vi "运维调试_采配水V3.vi"() -> ()   [LabVIEW 2016, in "PLC.lvlib"]
uses:
  PLC.lvlib
  <vilib>/Plasmionique/MB Master/MB_Master/MB_Master.lvclass
  <vilib>/Utility/miscctls.llb/LVPointTypeDef.ctl
  <vilib>/Plasmionique/MB Master/MB_Master_Serial/MB_Master_Serial.lvclass
  C:/Program Files (x86)/National Instruments/LabVIEW 2016/vi.lib/Plasmionique/MB Master/MB_Master/MB_Master.lvclass
  <vilib>/Instr/_visa.llb/VISA Configure Serial Port (Instr).vi
  <vilib>/NI/Modbus Library/API/Wrapper/Create TCP Slave.vi
  <vilib>/NI/Modbus Library/API/slave/Modbus Slave.lvclass
  <vilib>/Plasmionique/MB Master/MB Master.lvlib
  <vilib>/ptbypt/NI_PtbyPt.lvlib
  <vilib>/NI/Modbus Library/API/Wrapper/API Main.lvlib
panel:
  out "Registers":u16[](array[numeric])
  out "R124":i16 caption="加标回收配水时间"
  out "R44":i16
  in  "V14":bool
  in  "更新程序":bool
  out "R122":i16 caption="二级自来水清洗时间"
  out "R121":i16 caption="一级自来水清洗时间"
  out "R120":i16 caption="过滤自来水清洗时间"
  out "清洗次数":u16
  out "当前启动泵号":u16(ring) items=["1号泵", "2号泵"]
  out "R116":i16 caption="储水时间"
  in  "R113":u16(ring) caption="水箱储水水体" items=["自来水", "水样"]
  out "R112":i16 caption="二级水样池进样超时"
  in  "R111":u16(ring) caption="采配水型号" items=["常规版本", "高配版本"]
  out "数值 19":dbl
  out "数值 18":dbl
  out "数值 17":dbl
  out "数值 16":dbl
  out "数值 15":dbl
  out "数值 14":dbl
  out "数值 13":dbl
  out "数值 12":dbl
  out "数值 11":dbl
  out "数值 10":dbl
  out "数值 9":dbl
  out "数值 8":dbl
  out "数值 7":dbl
  out "数值 6":dbl
  out "数值 5":dbl
  out "数值 4":dbl
  out "数值 3":dbl
  out "数值 2":dbl
  out "数值":dbl
  in  "R118":u16(ring) caption="是否启用质控" items=["不启用质控", "启用质控"]
  out "压力传感器":dbl format="%#.2f"
  out "R110":i16 caption="过滤装置排液时间"
  in  "M4":bool
  in  "M3":bool
  in  "V13":bool
  in  "V12":bool
  in  "V1-R":bool
  in  "V1-G":bool
  in  "V11":bool
  in  "V10":bool
  in  "V9":bool
  in  "V8":bool
  in  "V7-R":bool
  in  "V7-G":bool
  out "X2":bool caption="X1"
  out "采配水版本号":string
  out "R117":i16 caption="清洗频次设定"
  out "通讯故障":bool
  in  "R100":u16(ring) caption="采水泵工作模式" items=["泵1单泵单管路", "泵2单泵单管路", "潜水泵双泵双管路", "自吸泵双泵双管路"]
  out "X11":bool caption="自来水检测_WA"
  out "X10":bool caption="废液报警_WLA"
  out "X9":bool caption="泵2过载报警_KM2"
  out "X8":bool caption="泵1过载报警_KM1"
  out "X7":bool caption="断电检测_DD"
  out "X6":bool caption="门禁开关_MJ"
  out "X5":bool caption="烟雾检测_YW"
  out "X4":bool caption="浸水检测_SJ"
  out "X3":bool caption="水流开关_JY"
  out "X1":bool
  out "X0":bool caption="采样池液位开关_YE1"
  out "R109":i16 caption="外部反冲洗时间"
  out "集成报警信息":string
  out "R108":i16 caption="进样超时时间"
  out "R107":i16 caption="进气时间"
  out "R106":i16 caption="排液时间"
  out "R105":i16 caption="常规模式配水时间"
  out "R104":i16 caption="过滤次数"
  out "R103":i16 caption="过滤配水时间"
  out "R102":i16 caption="一级沉淀时间"
  out "R101":i16 caption="管路润洗时间"
  out "R2":i16
  out "R1":i16
  out "多列列表框":i32(listbox)
  in  "V6":bool
  in  "V5":bool
  in  "V4":bool
  in  "V3":bool
  in  "V2":bool
  in  "M2":bool
  in  "M1":bool
  in  "返回":bool
  in  "参数设置":bool
  in  "单步启动":bool
  in  "启动":bool
  in  "停止":bool
  # "流程计时："
  # "s"
  # "压力传感器："
  # "MPa"
  # "二级液位开关低_Y2FD"
  # "二级液位开关高_YF2H"
  # "S"
  # "S"
  # "S"
  # "S"
  # "S"
  # "S"
  # "次"
  # "S"
  # "S"
  # "S"
  # "S"
  # "S"
  # "S"
  # "单步计时："
  # "s"
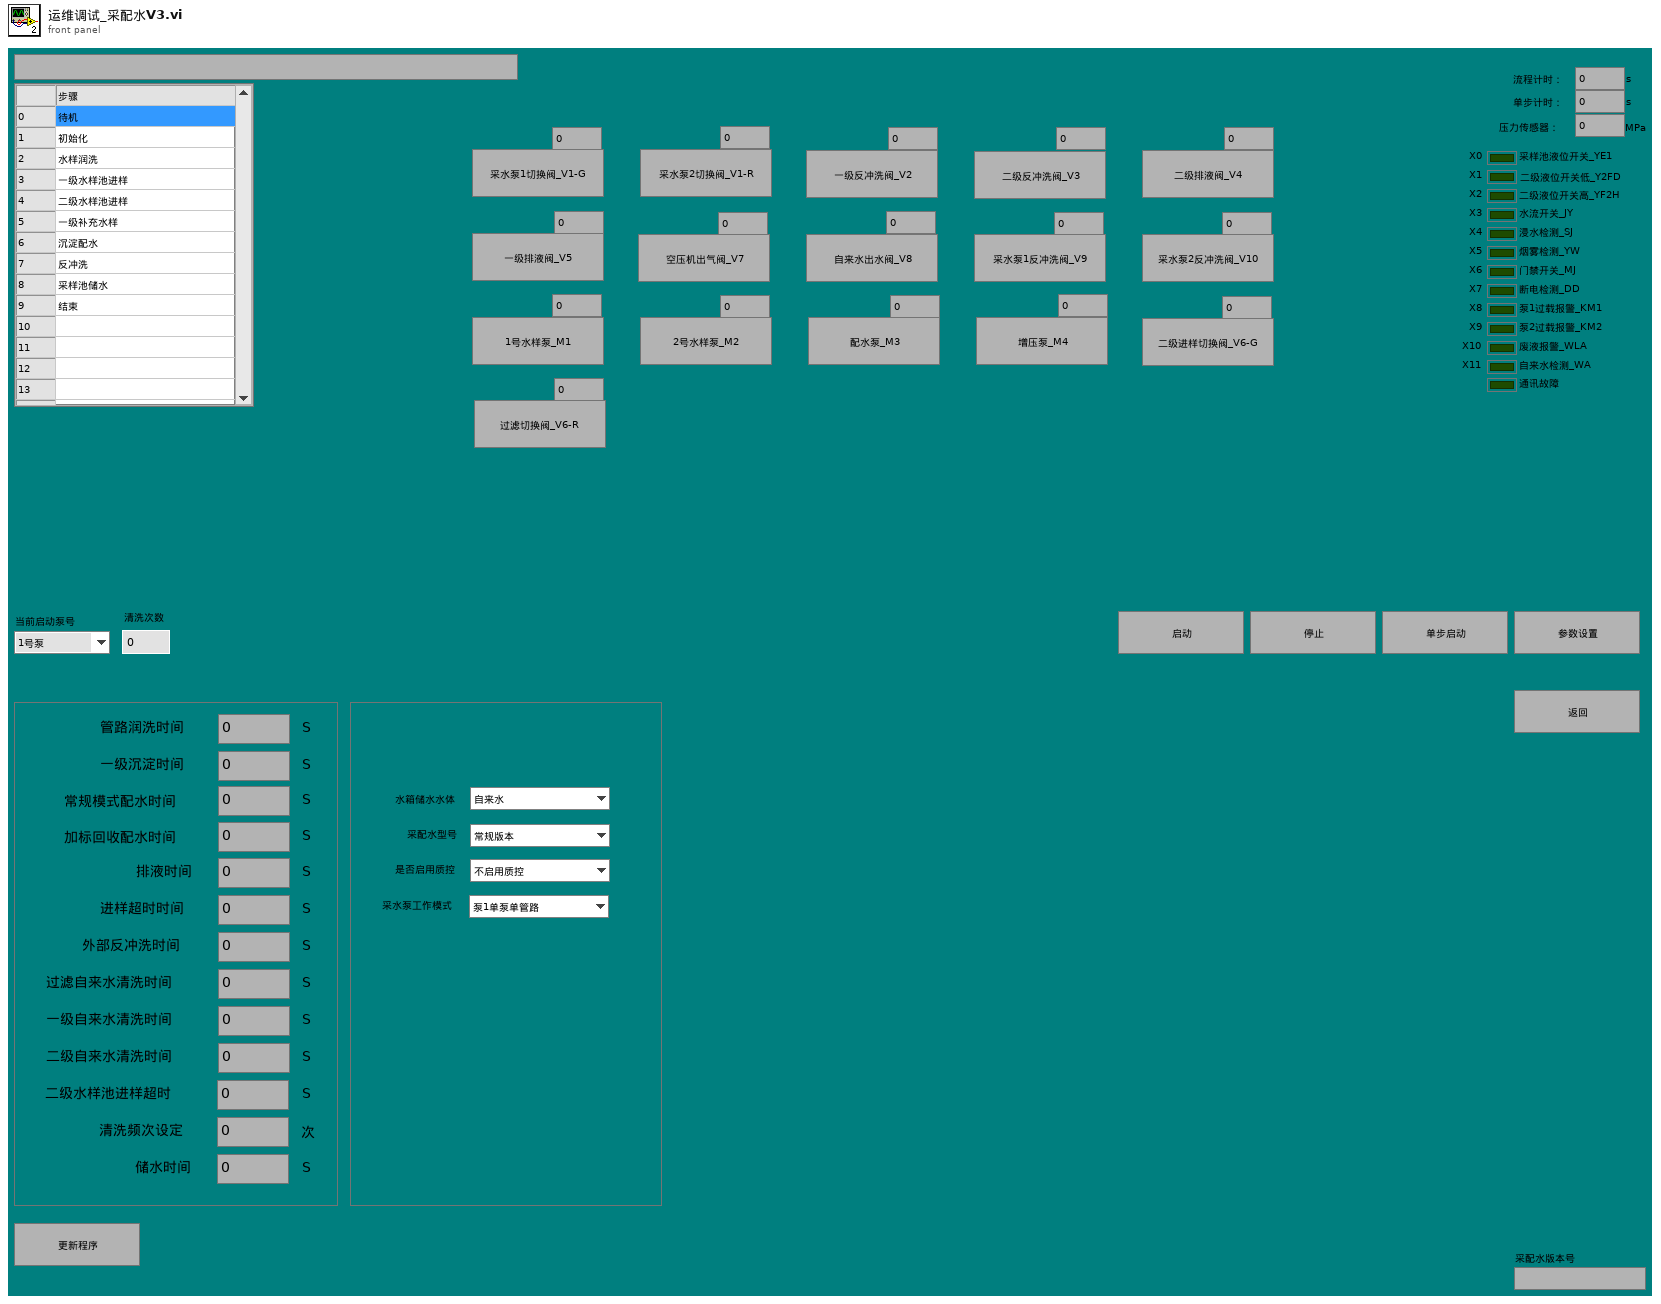
[diagram p1: front panel]
types:
  T1 = typedef "LVPointTypeDef.ctl" = cluster{"Horizontal":i16, "Vertical":i16}
  T2 = cluster{"命令":string, "数据":cluster{"starting address":u16, "holding register value":u16}}
  T3 = cluster{"时间标识":timestamp, "设备":string, "日志信息":string}
  T4 = cluster{"R0":i16, "R1":i16, "R2":i16, "R3":i16, "R4":i16, "R5":i16, "R6":i16, "R7":i16, "R8":i16, "R9":i16, "R10":i16, "R11":i16, "R12":i16, "R13":i16, "R14":i16, "R15":i16, "R16":i16, "R17":i16, "R18":i16, "R19":i16, "R20":i16, "R21":i16, "R22":i16, "R23":i16, "R24":i16, "R25":i16, "R26":i16, "R27":i16, "R28":i16, "R29":i16, "R30":i16, "R31":i16, "R32":i16, "R33":i16, "R34":i16, "R35":i16, "R36":i16, "R37":i16, "R38":i16, "R39":i16, "R40":i16, "R41":i16, "R42":i16, "R43":i16, "R44":i16, "R45":i16, "R46":i16, "R47":i16, "R48":i16, "R49":i16, "R50":i16, "R51":i16, "R52":i16, "R53":i16, "R54":i16, "R55":i16, "R56":i16}
  T5 = cluster{"seconds since 1Jan1904":timestamp, "table输入":string, string, "table输入":string}
  T6 = cluster{"时间标识":timestamp, "设备":string, "日志信息":string, "流程参数":string}
  T7 = cluster{"命令":string, cluster{"starting address":u16, "holding register value":u16}}
  T8 = cluster{"命令":string, "数据":cluster{"starting address":u16, "holding register values":u16[]}}
  T9 = cluster{"命令":string, "data":cluster{"starting address":u16, "coil values":bool[]}}
  T10 = cluster{"测试模式":enum16{"正常测试", "集成干预"}, "参数启用":cluster{"氨氮":bool, "总磷总氮":bool, "CODMn":bool, "CODcr":bool, "多参数":bool, "超标留样":bool, "总氮":bool}}
  T11 = enum32{"Bad", "Idle", "Run top level", "Running"}
  T12 = cluster{"baud rate (bps)":u32, "stop bits":u16, "parity":u16, "flow control":u16, "timeout":u32, "retries":i32}
  T13 = cluster{"starting address":u16, "holding register values":u16[]}
  T14 = cluster{"starting address":u16, "holding register value":u16}
  T15 = cluster{"starting address":u16, "coil values":bool[]}
  T16 = cluster{"Registers[0]":u16, "Registers[1]":u16, "Registers[2]":u16, "Registers[3]":u16, "Registers[4]":u16, "Registers[5]":u16, "Registers[6]":u16, "Registers[7]":u16, "Registers[8]":u16, "Registers[9]":u16, "Registers[10]":u16, "Registers[11]":u16, "Registers[12]":u16, "Registers[13]":u16, "Registers[14]":u16, "Registers[15]":u16, "Registers[16]":u16, "Registers[17]":u16, "Registers[18]":u16, "Registers[19]":u16, "Registers[20]":u16, "Registers[21]":u16, "Registers[22]":u16, "Registers[23]":u16, "Registers[24]":u16, "Registers[25]":u16, "Registers[26]":u16, "Registers[27]":u16, "Registers[28]":u16, "Registers[29]":u16, "Registers[30]":u16, "Registers[31]":u16, "Registers[32]":u16, "Registers[33]":u16, "Registers[34]":u16, "Registers[35]":u16, "Registers[36]":u16, "Registers[37]":u16, "Registers[38]":u16, "Registers[39]":u16, "Registers[40]":u16, "Registers[41]":u16, "Registers[42]":u16, "Registers[43]":u16, "Registers[44]":u16, "Registers[45]":u16, "Registers[46]":u16, "Registers[47]":u16, "Registers[48]":u16, "Registers[49]":u16, "Registers[50]":u16, "Registers[51]":u16, "Registers[52]":u16, "Registers[53]":u16, "Registers[54]":u16, "Registers[55]":u16, "Registers[56]":u16}
  T17 = cluster{"Registers[0]":u16, "Registers[1]":u16, "Registers[2]":u16, "Registers[3]":u16, "Registers[4]":u16, "Registers[5]":u16}
  T18 = cluster{"Registers[0]":u16, "Registers[1]":u16, "Registers[2]":u16, "Registers[3]":u16, "Registers[4]":u16, "Registers[5]":u16, "Registers[6]":u16, "Registers[7]":u16, "Registers[8]":u16, "Registers[9]":u16, "Registers[10]":u16, "Registers[11]":u16, "Registers[12]":u16, "Registers[13]":u16, "Registers[14]":u16, "Registers[15]":u16, "Registers[16]":u16, "Registers[17]":u16, "Registers[18]":u16, "Registers[19]":u16, "Registers[20]":u16, "Registers[21]":u16, "Registers[22]":u16, "Registers[23]":u16, "Registers[24]":u16}
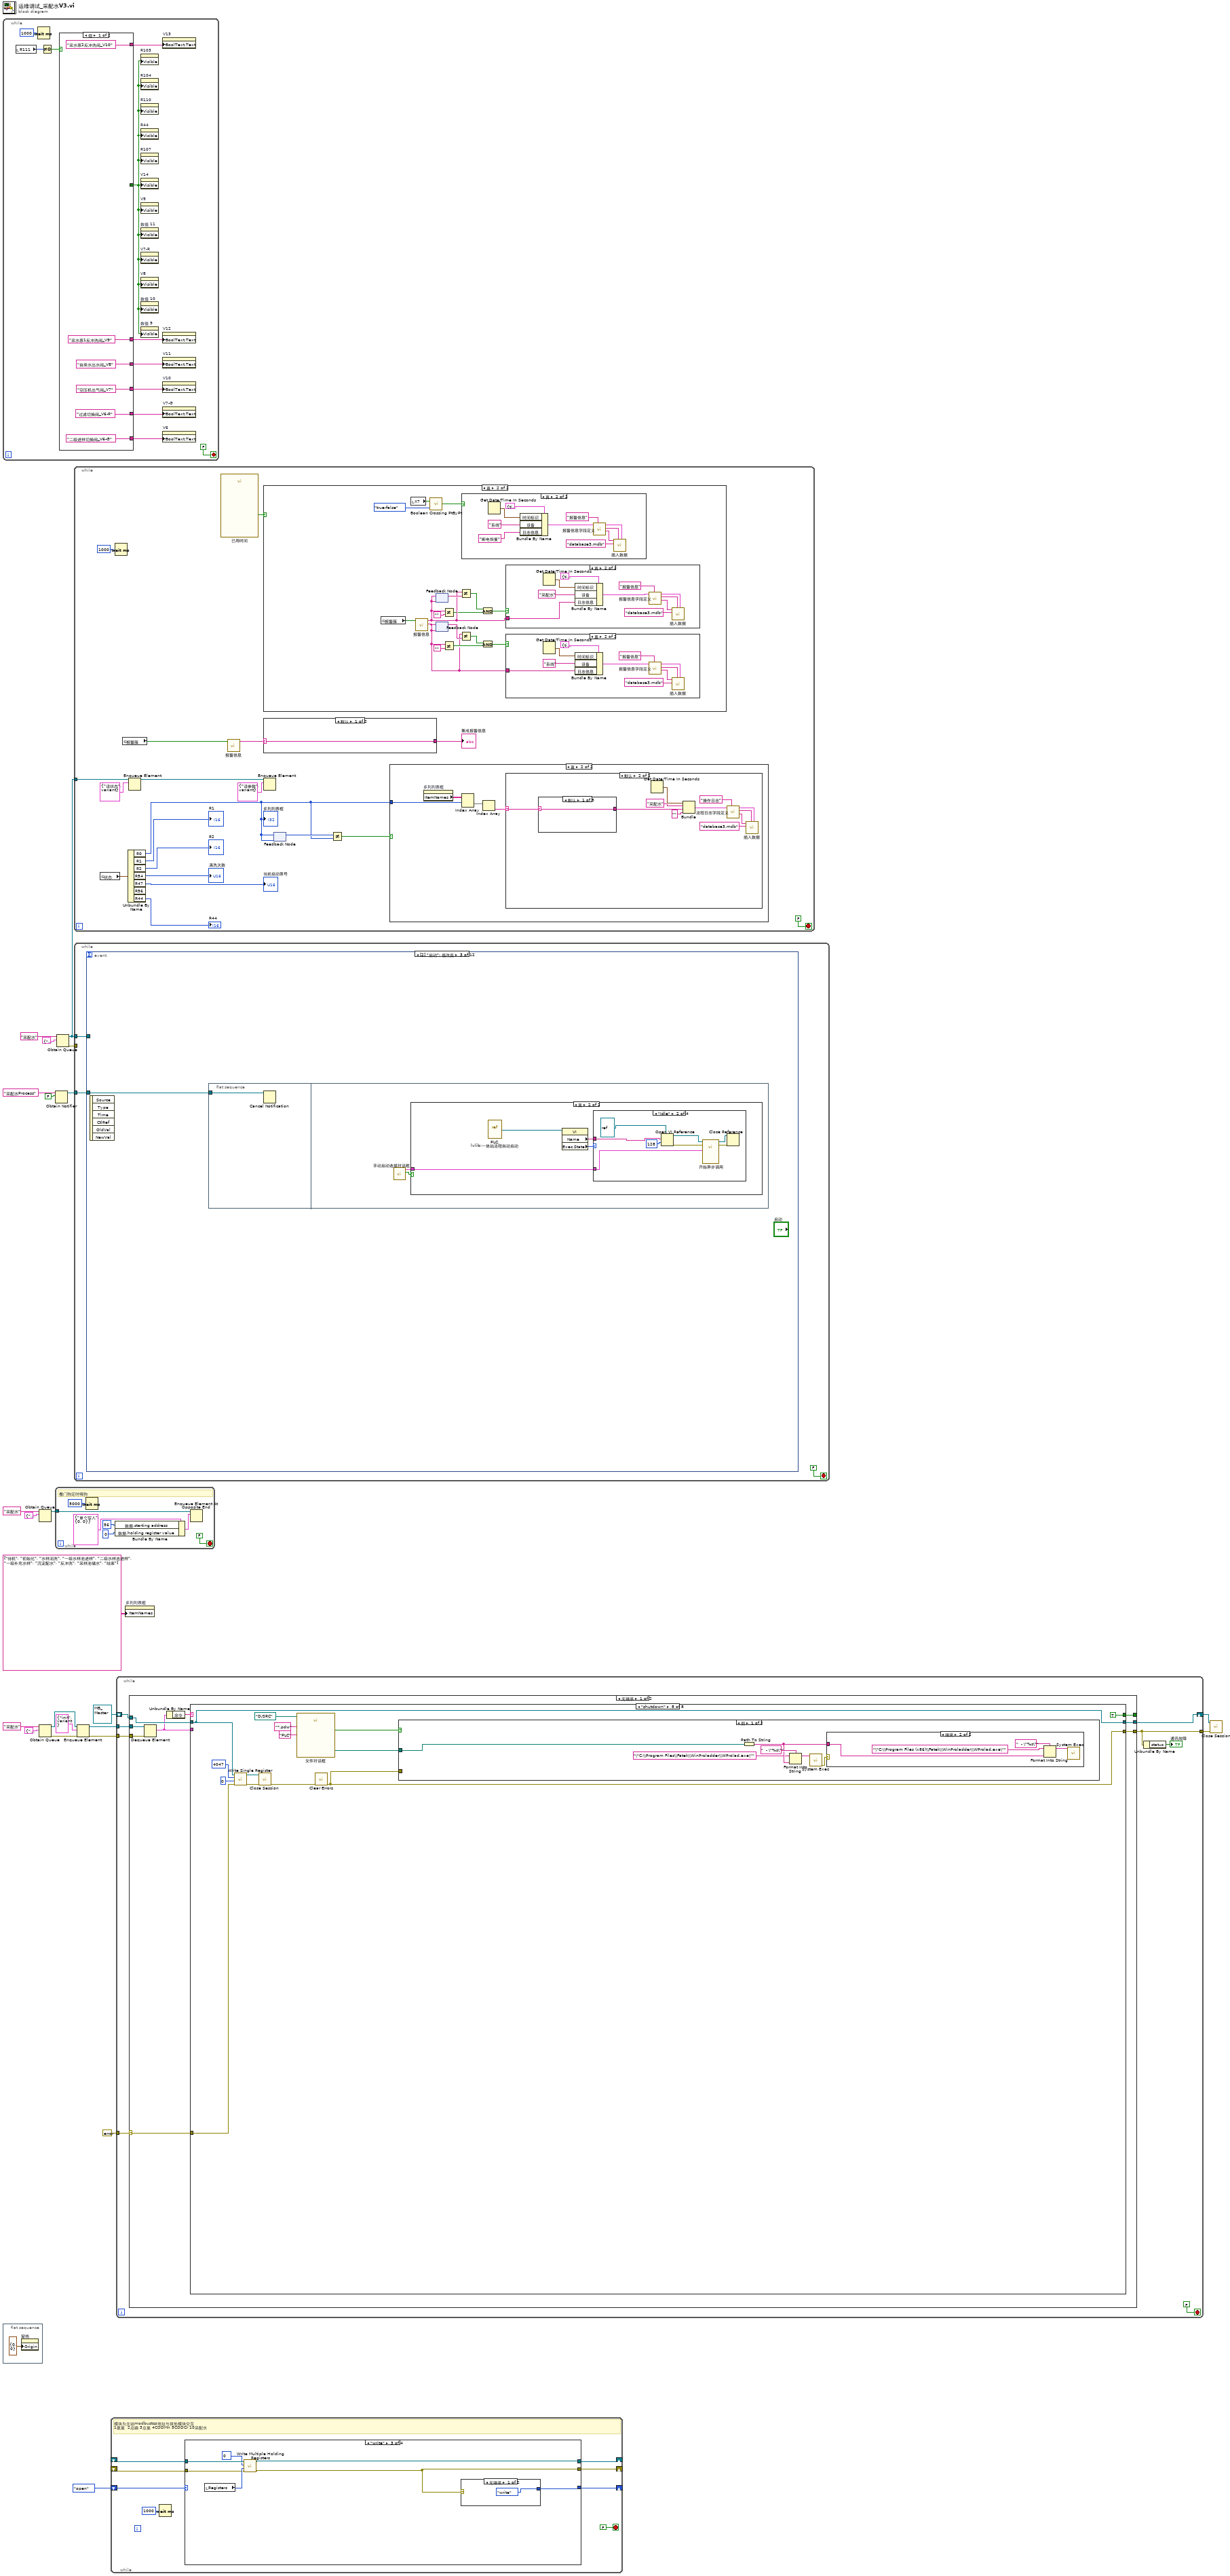
[diagram p0: block diagram]
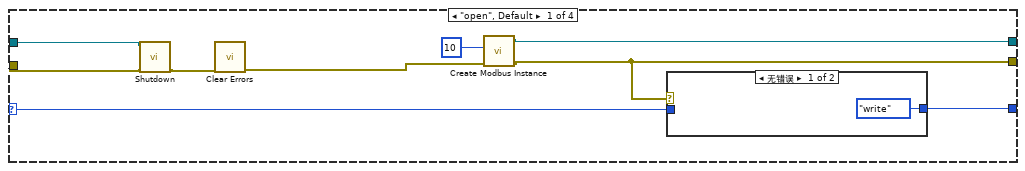
[diagram p2: hidden frame]
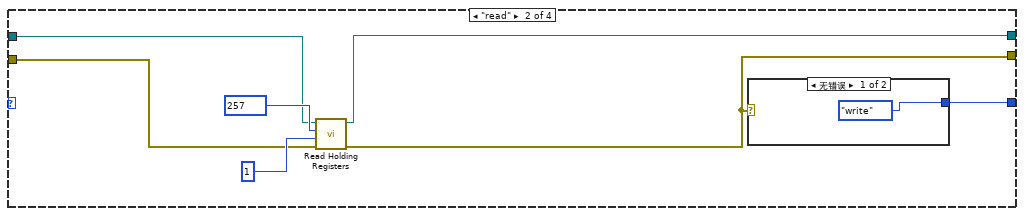
[diagram p4: hidden frame]
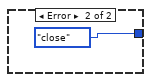
[diagram p5: hidden frame]
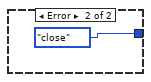
[diagram p6: hidden frame]
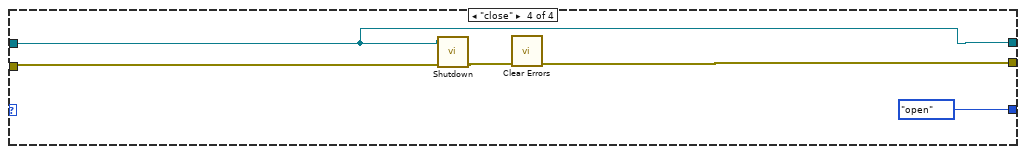
[diagram p7: hidden frame]
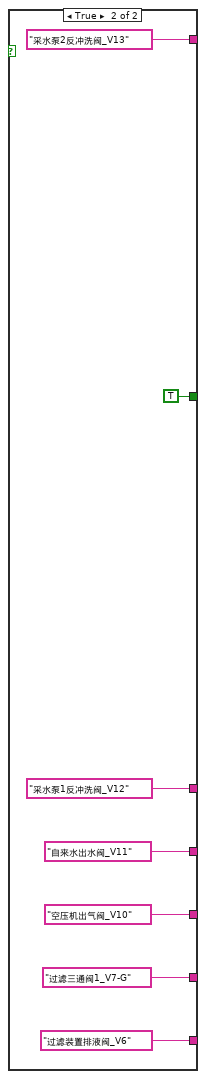
[diagram p8: hidden frame]
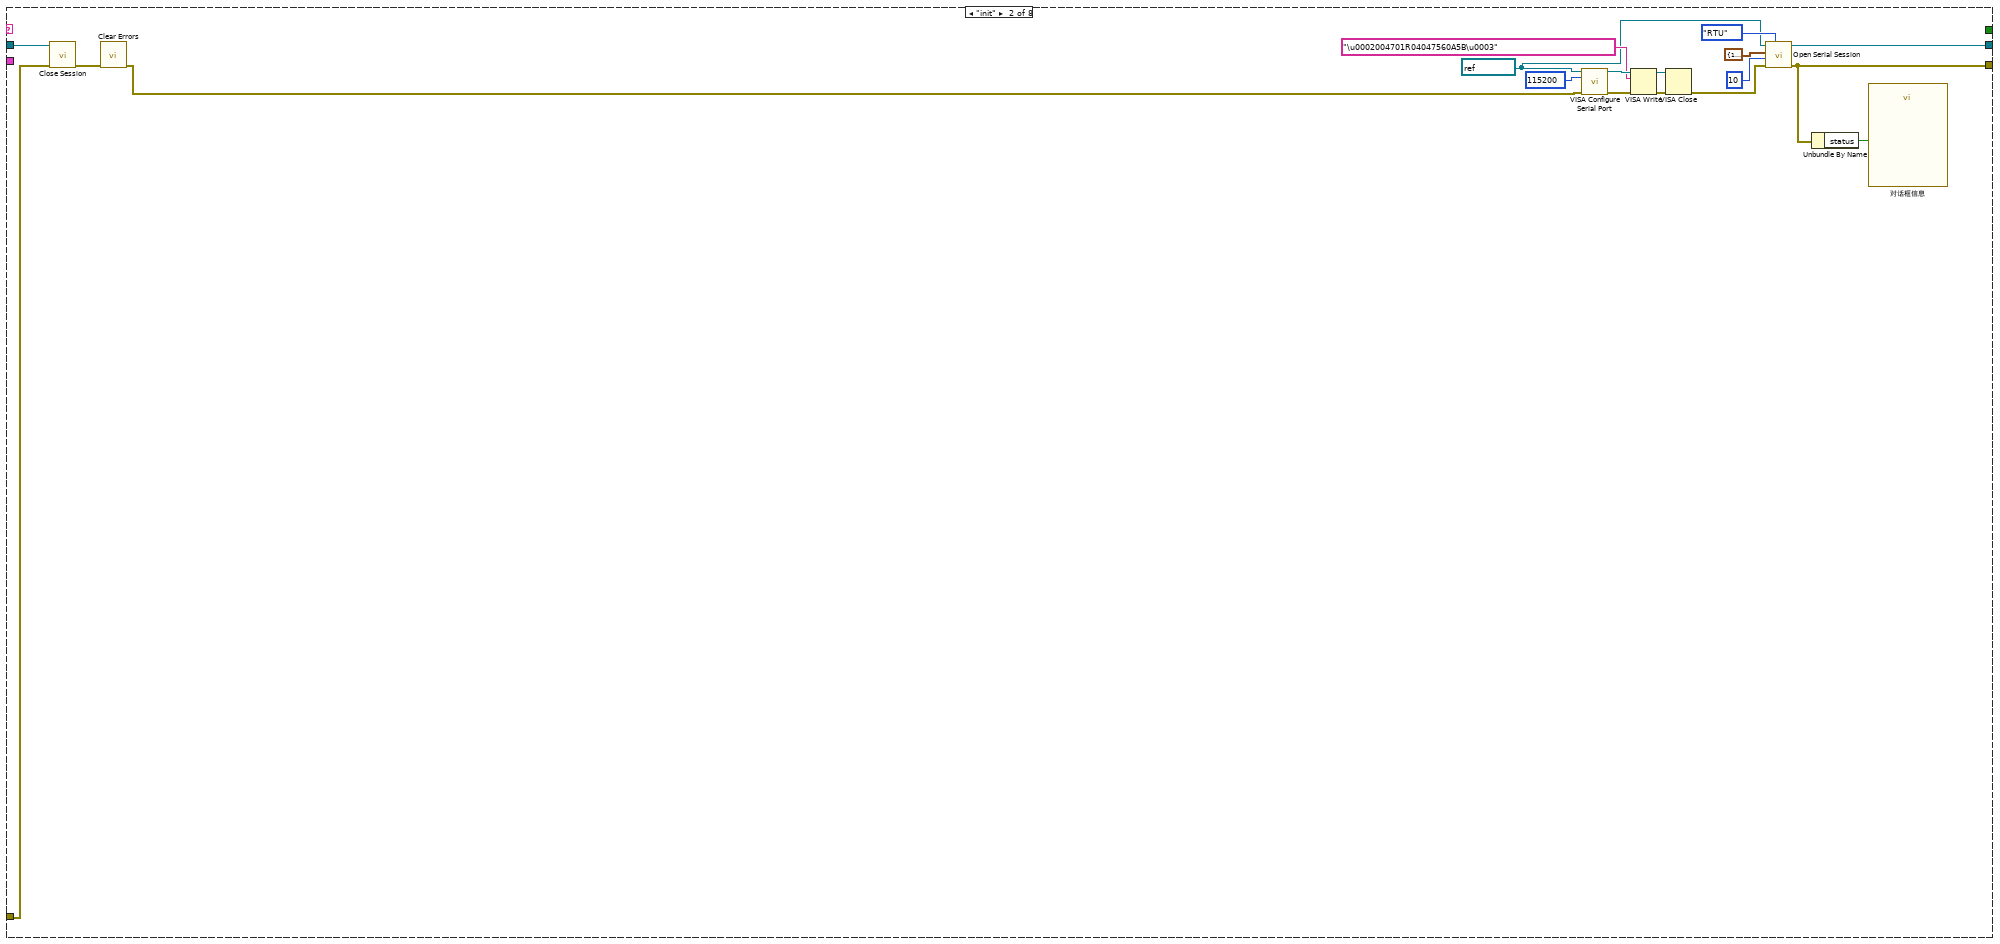
[diagram p10: hidden frame]
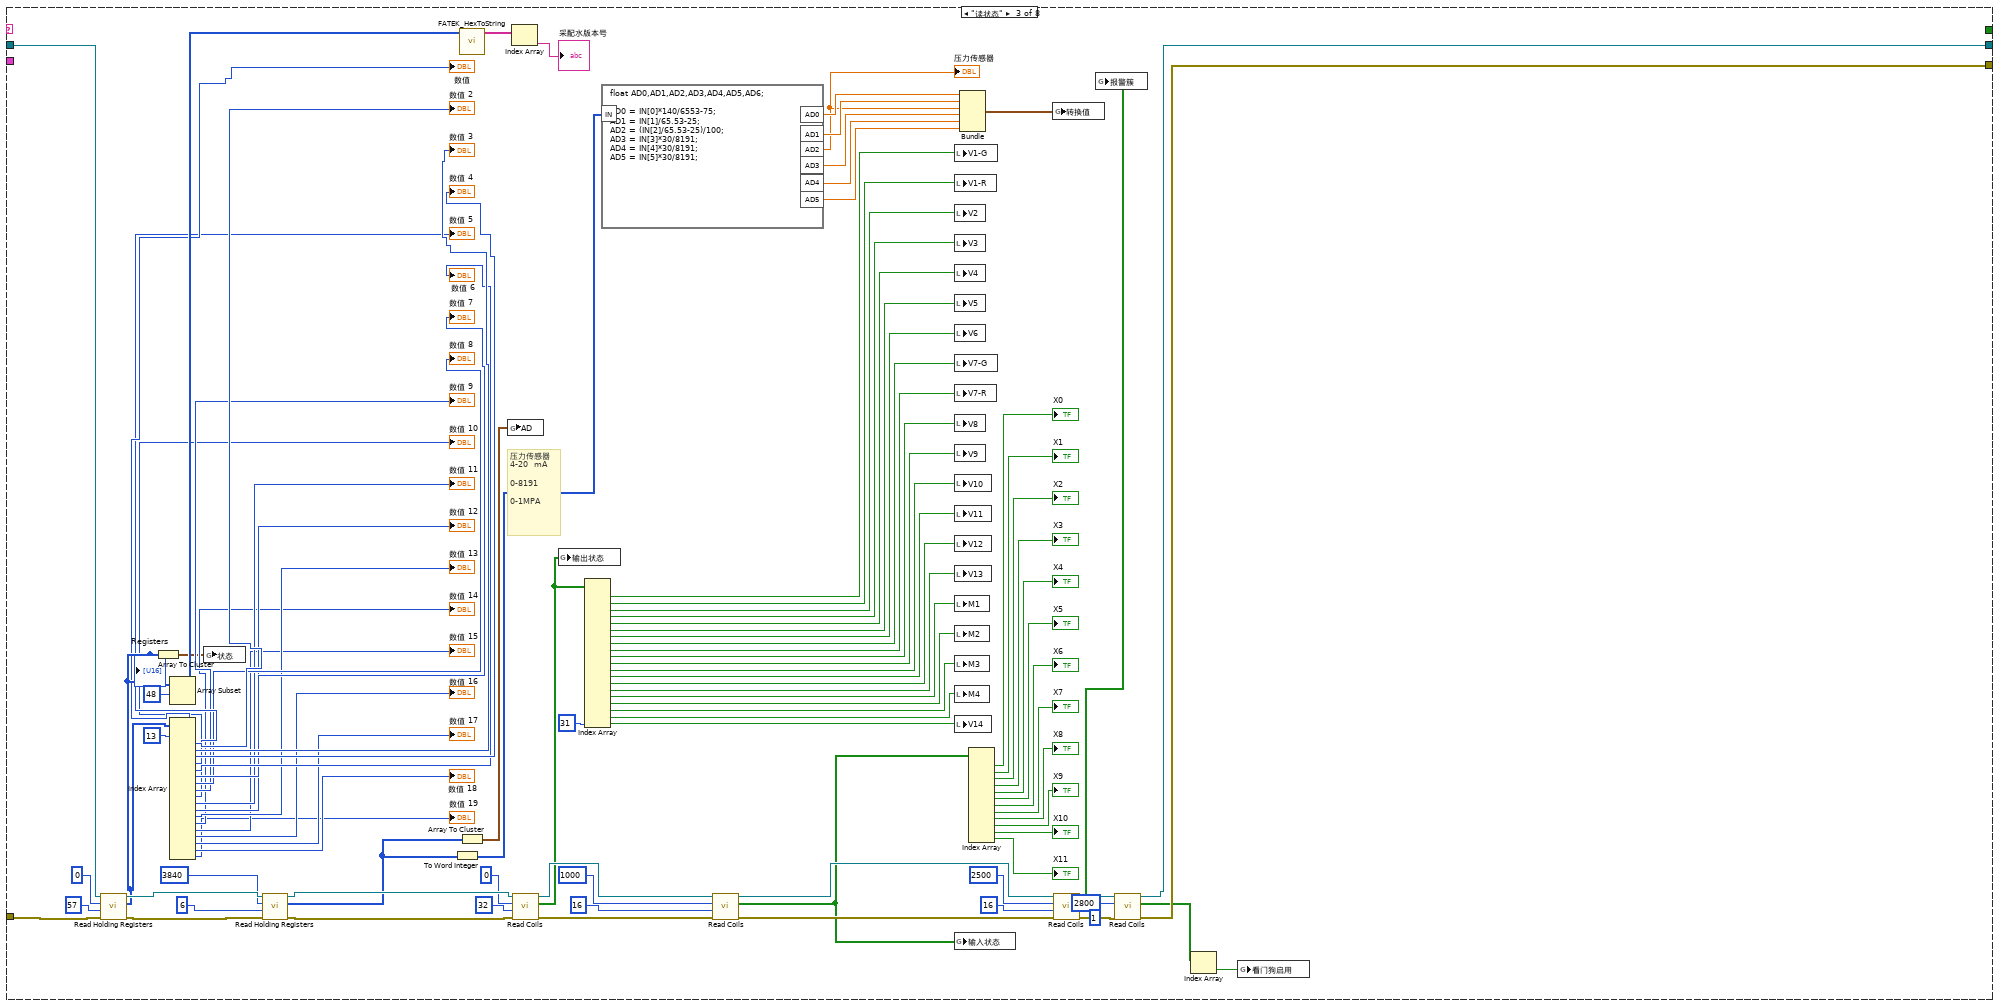
[diagram p11: hidden frame]
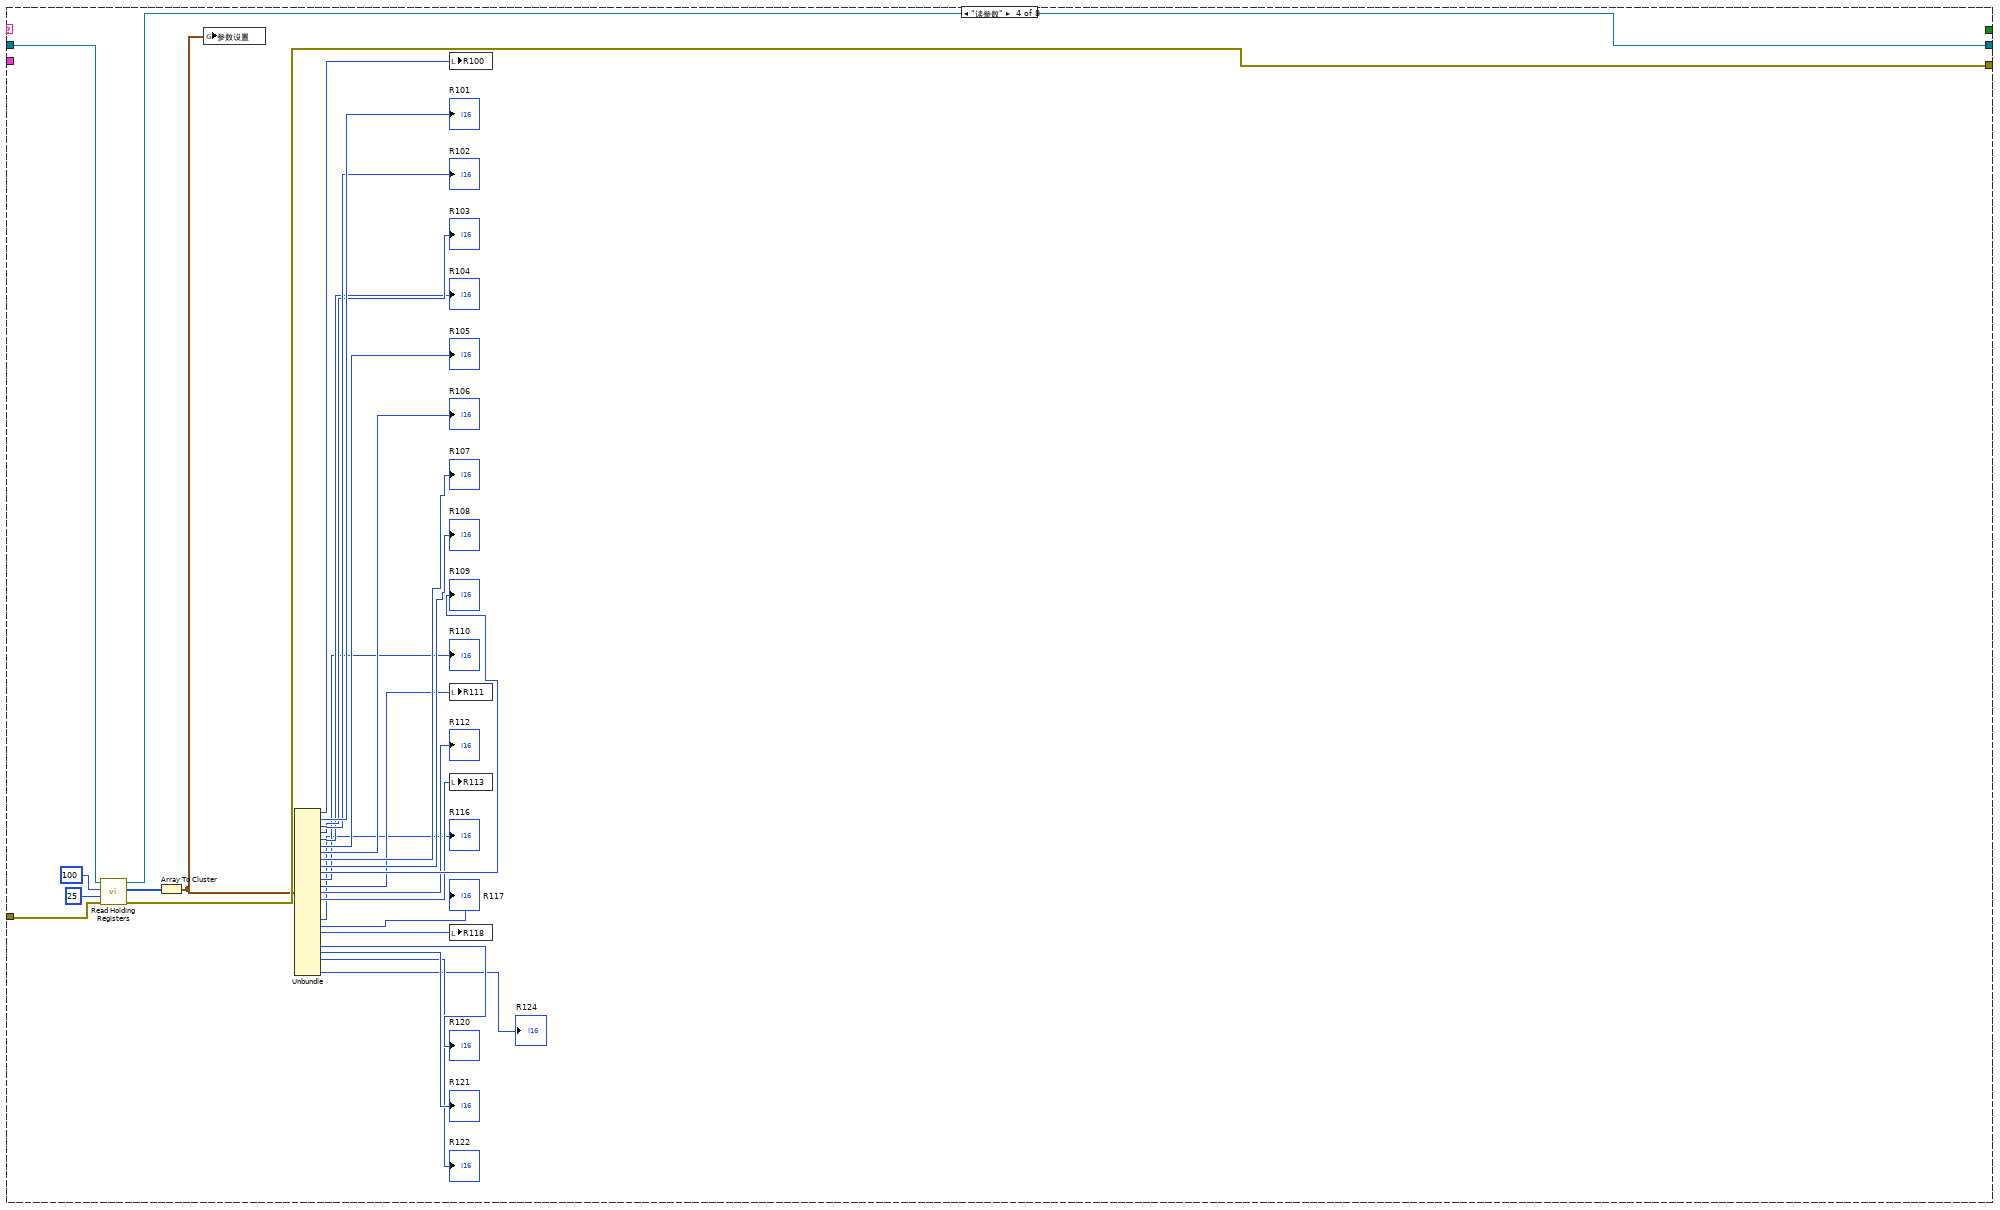
[diagram p12: hidden frame]
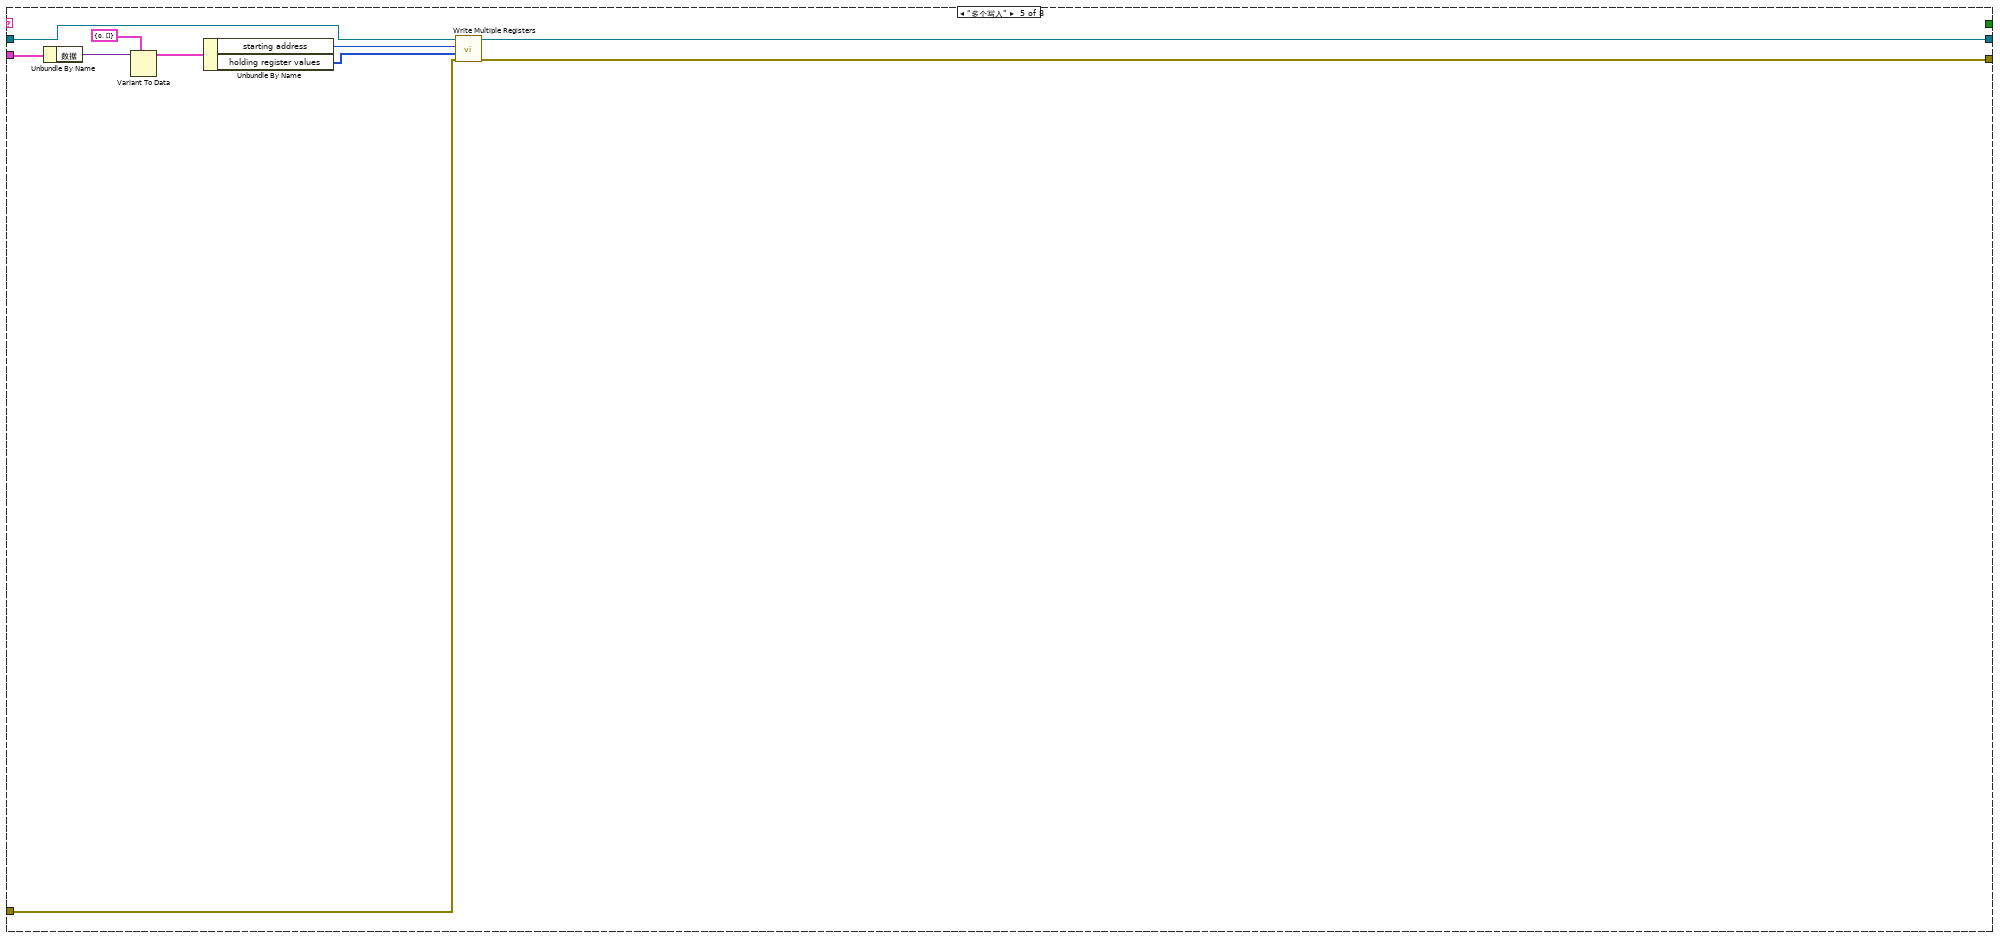
[diagram p13: hidden frame]
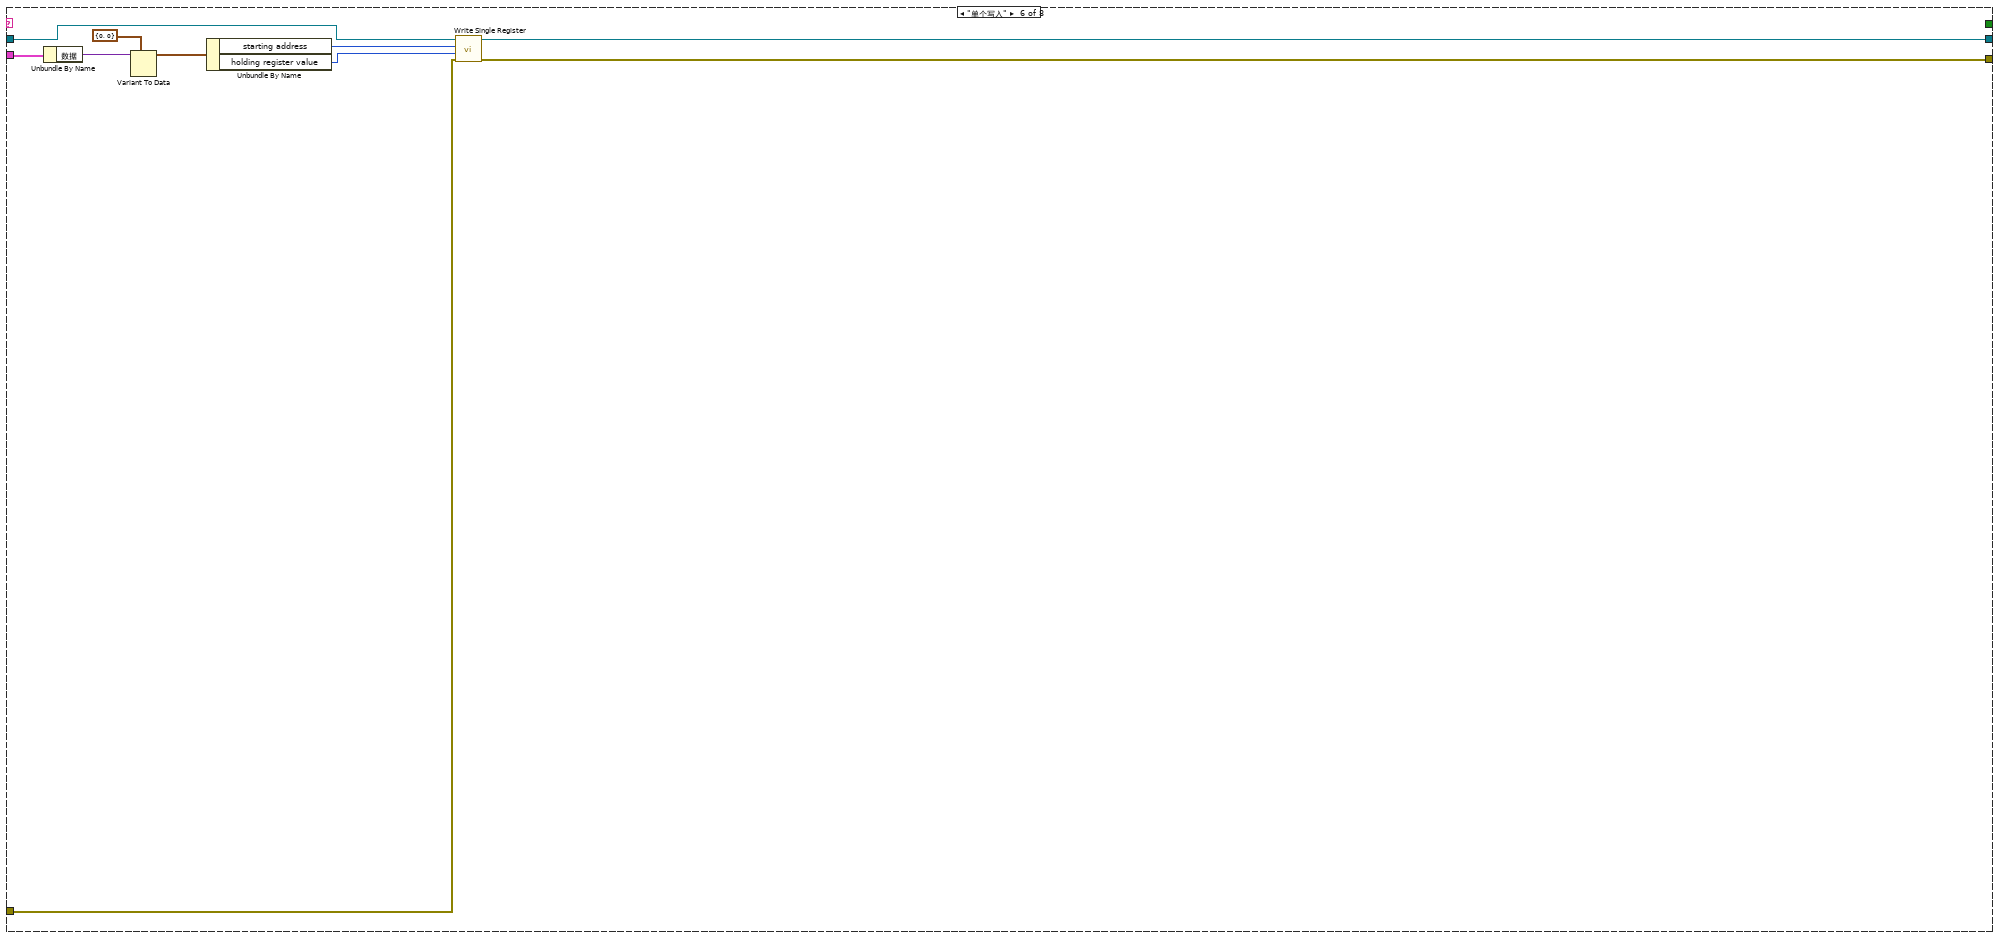
[diagram p14: hidden frame]
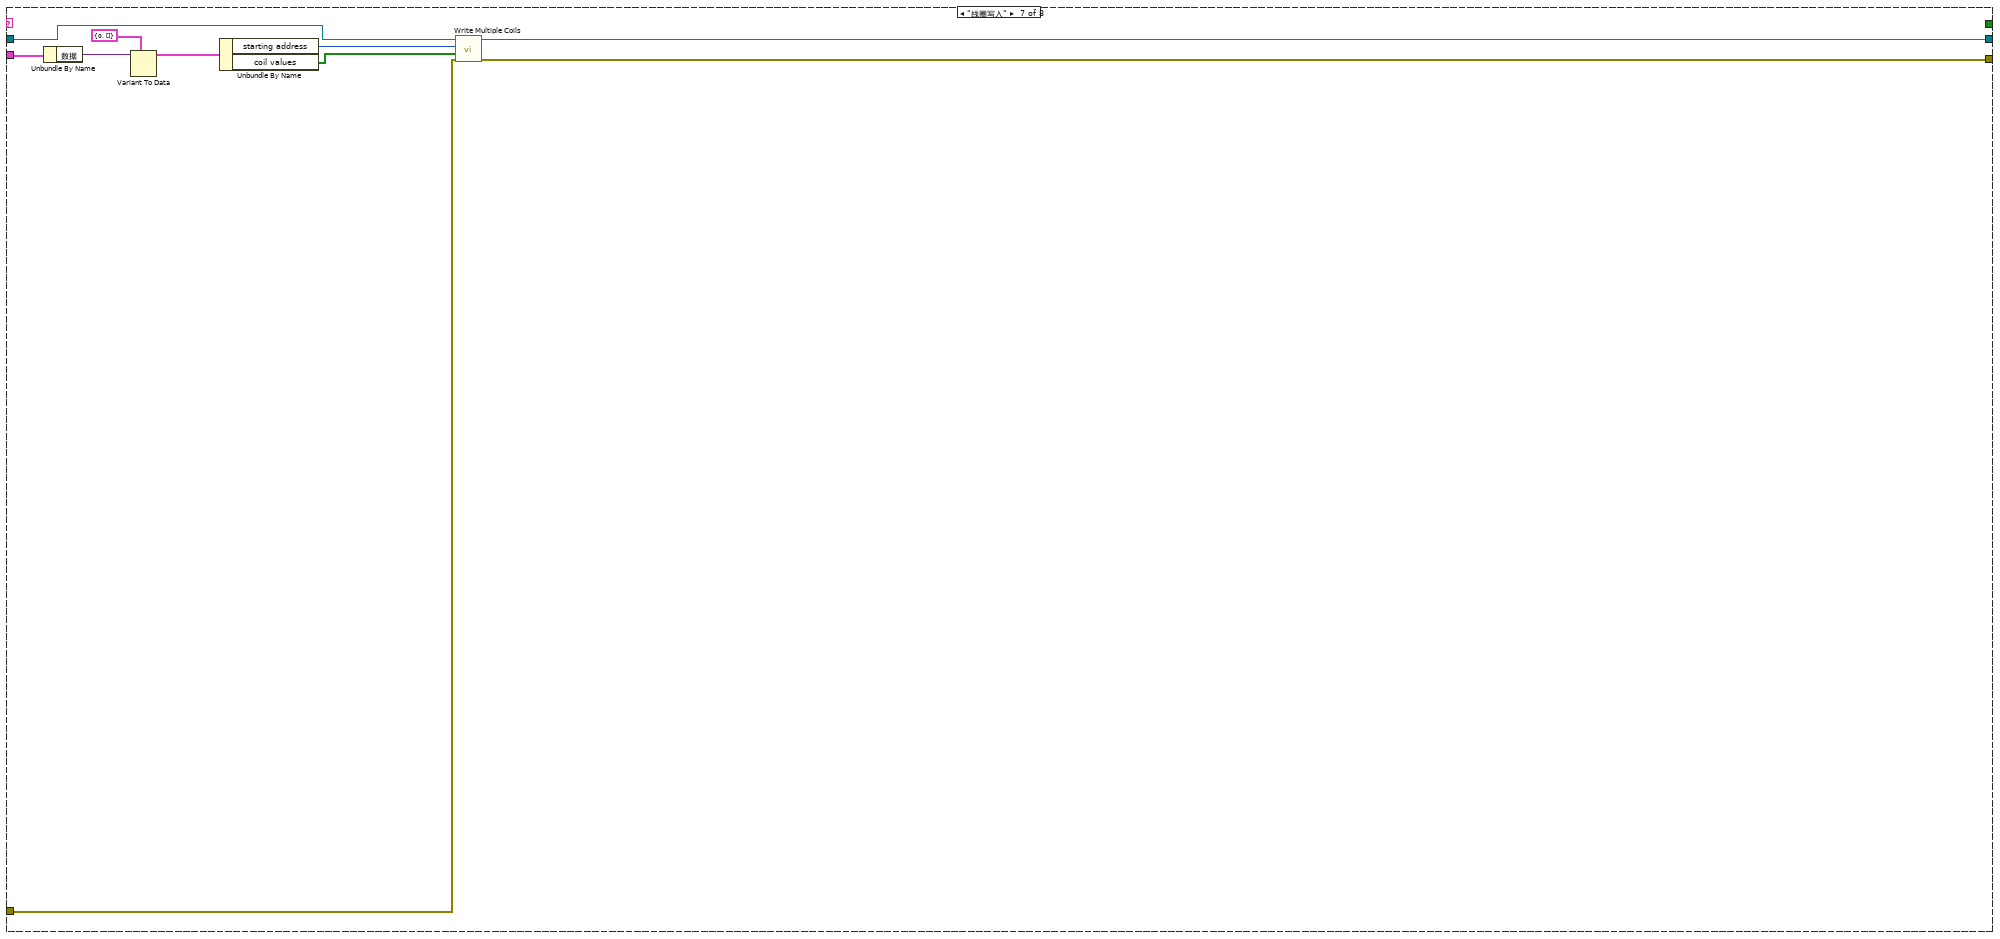
[diagram p15: hidden frame]
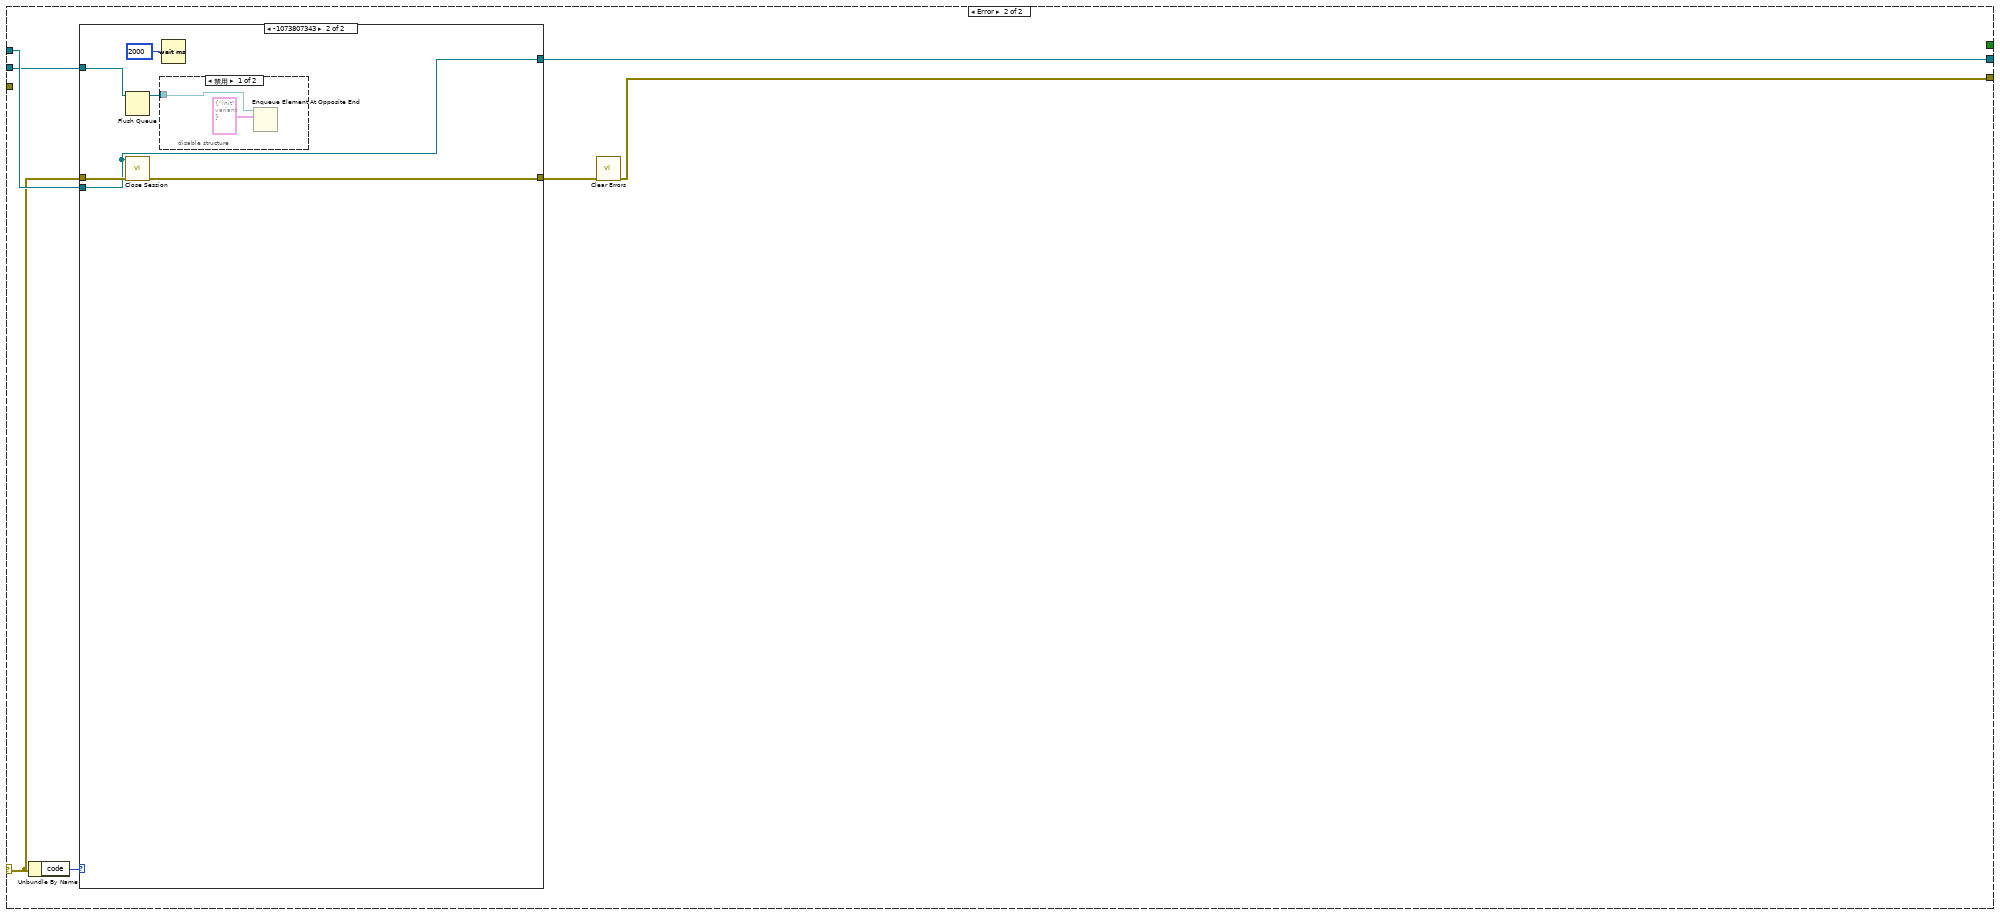
[diagram p18: hidden frame]
diagram:
  n1 = while {
    stop <- FALSE stop-if-true
    n2 = local read "R111"() -> (w33:u16)
    n3 = Wait (ms)(milliseconds to wait=u32 1000 ("等待时间（毫秒）")) -> ()  [unwired: 1 out]
    n4 = Not Equal To 0?(x=w33) -> (x != 0?=w32:bool)
    n5 = case shown="假" w32 {
      tunnel: [_ TRUE ("可见")] -> w24
      tunnel: ["二级进样切换阀_V6-G" ("布尔文本.文本") "过滤装置排液阀_V6" ("布尔文本.文本")] -> w30
      tunnel: ["过滤切换阀_V6-R" ("布尔文本.文本") "过滤三通阀1_V7-G" ("布尔文本.文本")] -> w29
      tunnel: ["空压机出气阀_V7" ("布尔文本.文本") "空压机出气阀_V10" ("布尔文本.文本")] -> w28
      tunnel: ["自来水出水阀_V8" ("布尔文本.文本") "自来水出水阀_V11" ("布尔文本.文本")] -> w27
      tunnel: ["采水泵1反冲洗阀_V9" ("布尔文本.文本") "采水泵1反冲洗阀_V12" ("布尔文本.文本")] -> w26
      tunnel: ["采水泵2反冲洗阀_V10" ("布尔文本.文本") "采水泵2反冲洗阀_V13" ("布尔文本.文本")] -> w25
      frame False {
      }
      frame True {
      }
    }
    n6 = property on="R103" class="DigNum (严格)"("Visible"=w24) -> ()  [unwired: 2 in, 2 out]
    n7 = property on="R104" class="DigNum (严格)"("Visible"=w24) -> ()  [unwired: 2 in, 2 out]
    n8 = property on="R110" class="DigNum (严格)"("Visible"=w24) -> ()  [unwired: 2 in, 2 out]
    n9 = property on="R44" class="DigNum (严格)"("Visible"=w24) -> ()  [unwired: 2 in, 2 out]
    n10 = property on="R107" class="DigNum (严格)"("Visible"=w24) -> ()  [unwired: 2 in, 2 out]
    n11 = property on="V14" class="Bool (严格)"("Visible"=w24) -> ()  [unwired: 2 in, 2 out]
    n12 = property on="V9" class="Bool (严格)"("Visible"=w24) -> ()  [unwired: 2 in, 2 out]
    n13 = property on="数值 11" class="DigNum (严格)"("Visible"=w24) -> ()  [unwired: 2 in, 2 out]
    n14 = property on="V7-R" class="Bool (严格)"("Visible"=w24) -> ()  [unwired: 2 in, 2 out]
    n15 = property on="V8" class="Bool (严格)"("Visible"=w24) -> ()  [unwired: 2 in, 2 out]
    n16 = property on="数值 10" class="DigNum (严格)"("Visible"=w24) -> ()  [unwired: 2 in, 2 out]
    n17 = property on="数值 9" class="DigNum (严格)"("Visible"=w24) -> ()  [unwired: 2 in, 2 out]
    n18 = property on="V13" class="Bool (严格)"("BoolText.Text"=w25) -> ()  [unwired: 2 in, 2 out]
    n19 = property on="V12" class="Bool (严格)"("BoolText.Text"=w26) -> ()  [unwired: 2 in, 2 out]
    n20 = property on="V11" class="Bool (严格)"("BoolText.Text"=w27) -> ()  [unwired: 2 in, 2 out]
    n21 = property on="V10" class="Bool (严格)"("BoolText.Text"=w28) -> ()  [unwired: 2 in, 2 out]
    n22 = property on="V7-G" class="Bool (严格)"("BoolText.Text"=w29) -> ()  [unwired: 2 in, 2 out]
    n23 = property on="V6" class="Bool (严格)"("BoolText.Text"=w30) -> ()  [unwired: 2 in, 2 out]
  }
  n24 = flat-sequence {
    frame #0 {
      n25 = property on="窗格" class="Pane"("Origin"=T1 {"Horizontal"=0, "Vertical"=0} ("原点")) -> ()  [unwired: 2 in, 2 out]
    }
  }
  n26 = Obtain Queue(name (unnamed)="采配水" ("名称（未命名）"), element data type=cluster{"命令":string, "数据":variant} {"命令"="", "数据"=variant}) -> (queue out=w2:refnum<queue>)  [unwired: 3 in, 2 out]
  n27 = Obtain Queue(name (unnamed)="采配水" ("名称（未命名）"), element data type=cluster{"命令":string, "数据":variant} {"命令"="", "数据"=variant}) -> (queue out=w13:refnum<queue>, error out=w12:errorcluster)  [unwired: 3 in, 1 out]
  n28 = Obtain Notifier(name (unnamed)="采配水Process" ("名称（未命名）"), notification data type=FALSE) -> (notifier out=w16:refnum<notifier>)  [unwired: 2 in, 2 out]
  n29 = while {
    tunnel: w2 -> [w53]
    stop <- FALSE stop-if-true
    # "看门狗定时喂狗"
    n30 = Wait (ms)(milliseconds to wait=u32 5000 ("等待时间（毫秒）")) -> ()  [unwired: 1 out]
    n31 = Bundle By Name(cluster=T2 {"命令"="单个写入", "数据"={"starting address"=0, "holding register value"=0}} ("元素"), "数据.starting address"=u16 56, "数据.holding register value"=u16 0) -> (w54:T2)
    n32 = Enqueue Element At Opposite End(queue=w53, element=w54) -> ()  [unwired: 2 in, 3 out]
  }
  n33 = Obtain Queue(name (unnamed)="采配水" ("名称（未命名）"), element data type=cluster{"命令":string, "数据":variant} {"命令"="", "数据"=variant}) -> (queue out=w20:refnum<queue>, error out=w21:errorcluster)  [unwired: 3 in, 1 out]
  n34 = while {
    tunnel: w20 -> [w73]
    stop <- FALSE stop-if-true
    n35 = global read "采配水全局变量.vi" "状态"() -> (w71:T4)
    n36 = Wait (ms)(milliseconds to wait=u32 1000 ("等待时间（毫秒）")) -> ()  [unwired: 1 out]
    n37 = global read "采配水全局变量.vi" "报警簇"() -> (w67:bool[])
    n38 = Unbundle By Name(w71) -> ("R0"=w60:i16, "R1"=→"R1":i16, "R2"=→"R2":i16, "R54"=→"清洗次数":i16, "R47"=→"当前启动泵号":i16, "R44"=→"R44":i16)  [unwired: 1 out]
    "多列列表框" <- w60
    n39 = Enqueue Element(queue=w73, element=cluster{"命令":string, "数据":variant} {"命令"="读状态", "数据"=variant} ("元素")) -> (queue out=w62:refnum<queue>)  [unwired: 2 in, 2 out]
    n40 = call "已用时间"() -> ("Time has Elapsed"=w65:bool)  [unwired: 12 in, 7 out]
    n41 = call "报警信息.vi"("报警簇"=w67) -> ("采配水报警信息"=w59:string)  [unwired: 9 in, 1 out]
    n42 = case shown="真" w65 {
      frame False {
      }
      frame True {
        n43 = global read "采配水全局变量.vi" "报警簇"() -> (w90:bool[])
        n44 = local read "X7"() -> (w77:bool)
        n45 = call "报警信息.vi"("报警簇"=w90) -> ("系统报警信息"=w79:string, "采配水报警信息"=w86:string)  [unwired: 9 in]
        n46 = call <vilib>:"Boolean Crossing PtByPt.vi"("direction"=enum16{"either", "false-true", "true-false"}."true-false", "input"=w77) -> ("crossing"=w75:bool)  [unwired: 1 in]
        n47 = feedback #1(w86) -> (w89:string)
        n48 = feedback-in #1(w86) -> ()
        n49 = feedback #2(w79) -> (w80:string)
        n50 = feedback-in #2(w79) -> ()
        n51 = Not Equal?(x=w86, y="") -> (x != y?=w84:bool)
        n52 = Not Equal?(x=w79, y="") -> (x != y?=w83:bool)
        n53 = Not Equal?(x=w86, y=w89) -> (x != y?=w88:bool)
        n54 = Not Equal?(x=w79, y=w80) -> (x != y?=w81:bool)
        n55 = case shown="真" w75 {
          frame False {
          }
          frame True {
            n56 = Get Date/Time In Seconds() -> (seconds since 1Jan1904=w99:timestamp)
            n57 = Bundle By Name(cluster=T3 {"时间标识"=timestamp(0 s since 1904-01-01), "设备"="", "日志信息"=""} ("data in"), "时间标识"=w99, "设备"="系统", "日志信息"="断电恢复") -> (w98:T3)
            n58 = call "报警信息字段定义.vi"("table输入"="报警信息", "data in"=w98) -> ("table输出"=w94:string, "columns"=w93:string[], "data out"=w92:T3)  [unwired: 7 in]
            n59 = call "插入数据.vi"("data"=w92, "columns"=w93, "database"="database3.mdb", "table"=w94) -> ()  [unwired: 7 in, 1 out]
          }
        }
        n60 = And(x=w88, y=w84) -> (x .and. y?=w87:bool)
        n61 = And(x=w81, y=w83) -> (x .and. y?=w78:bool)
        n62 = case shown="真" w87 {
          tunnel: w86 -> [_ w111]
          frame False {
          }
          frame True {
            n63 = Get Date/Time In Seconds() -> (seconds since 1Jan1904=w113:timestamp)
            n64 = Bundle By Name(cluster=T3 {"时间标识"=timestamp(0 s since 1904-01-01), "设备"="", "日志信息"=""} ("data in"), "时间标识"=w113, "设备"="采配水", "日志信息"=w111) -> (w114:T3)
            n65 = call "报警信息字段定义.vi"("table输入"="报警信息", "data in"=w114) -> ("table输出"=w118:string, "columns"=w119:string[], "data out"=w120:T3)  [unwired: 7 in]
            n66 = call "插入数据.vi"("data"=w120, "columns"=w119, "database"="database3.mdb", "table"=w118) -> ()  [unwired: 7 in, 1 out]
          }
        }
        n67 = case shown="真" w78 {
          tunnel: w79 -> [_ w101]
          frame False {
          }
          frame True {
            n68 = Get Date/Time In Seconds() -> (seconds since 1Jan1904=w103:timestamp)
            n69 = Bundle By Name(cluster=T3 {"时间标识"=timestamp(0 s since 1904-01-01), "设备"="", "日志信息"=""} ("data in"), "时间标识"=w103, "设备"="系统", "日志信息"=w101) -> (w104:T3)
            n70 = call "报警信息字段定义.vi"("table输入"="报警信息", "data in"=w104) -> ("table输出"=w108:string, "columns"=w109:string[], "data out"=w110:T3)  [unwired: 7 in]
            n71 = call "插入数据.vi"("data"=w110, "columns"=w109, "database"="database3.mdb", "table"=w108) -> ()  [unwired: 7 in, 1 out]
          }
        }
      }
    }
    n72 = case shown="默认" w59 {
      selector: w59 -> [w121 _]
      tunnel: [w121 w122] -> w66
      frame Default {
      }
      frame "" {
        n73 = global read "采配水全局变量.vi" "运行状态显示"() -> (w122:string)
      }
    }
    "集成报警信息" <- w66
    n74 = Enqueue Element(queue=w62, element=cluster{"命令":string, "数据":variant} {"命令"="读参数", "数据"=variant} ("元素")) -> ()  [unwired: 2 in, 3 out]
    n75 = feedback-in #3(w60) -> ()
    n76 = feedback #3(w60) -> (w61:i16)
    n77 = Not Equal?(x=w61, y=w60) -> (x != y?=w68:bool)
    n78 = case shown="真" w68 {
      tunnel: w60 -> [_ w125]
      frame False {
      }
      frame True {
        n79 = property on="多列列表框" class="MCListbox (严格)"() -> ("ItemNames"=w126:string[][])  [unwired: 2 in, 2 out]
        n80 = Index Array(array=w126, index (row)=w125) -> (element=w124:string[])  [unwired: 1 in]
        n81 = Index Array(array=w124) -> (element=w123:string)  [unwired: 1 in]
        n82 = case shown="默认" w123 {
          selector: w123 -> [_ w128]
          frame "待机" {
          }
          frame Default {
            n83 = case shown="默认" w128 {
              selector: w128 -> [w138 _ _]
              tunnel: [w138 "-->>启动" "-->>结束"] -> w127
              frame Default {
              }
              frame "初始化" {
              }
              frame "结束" {
              }
            }
            n84 = Get Date/Time In Seconds() -> (seconds since 1Jan1904=w132:timestamp)
            n85 = Bundle("seconds since 1Jan1904"=w132, "table输入"="采配水", w127, "table输入"="") -> (w130:T5)  [unwired: 1 in]
            n86 = call "流程日志字段定义.vi"("table输入"="操作日志", "data in"=w130) -> ("table输出"=w135:string, "columns"=w136:string[], "data out"=w137:T6)  [unwired: 7 in]
            n87 = call "插入数据.vi"("data"=w137, "columns"=w136, "database"="database3.mdb", "table"=w135) -> ()  [unwired: 7 in, 1 out]
          }
        }
      }
    }
  }
  n88 = while {
    tunnel: w20 -> [w142]
    tunnel: w21 -> [_]
    tunnel: w16 -> [w141]
    stop <- FALSE stop-if-true
    n89 = event shown="[2] \"启动\": 值改变" {
      selector: _ -> [_ _ _ _ _ _ _ _ _ _ _ _]
      dyn-events: _ -> [_ _ _ _ _ _ _ _ _ _ _ _]
      timeout: _ -> [_ _ _ _ _ _ _ _ _ _ _ _]
      tunnel: w142 -> [_ w146 _ w168 w187 w196 w201 _ _ _ w235 w239]
      tunnel: w141 -> [_ w145 w148 _ _ _ _ _ _ _ _ _]
      event Timeout {
        n90 = event-data() -> ()  [unwired: 1 in, 3 out]
      }
      event "停止": Value Change {
        n91 = event-data() -> ()  [unwired: 1 in, 6 out]
        n92 = Send Notification(notification=TRUE ("通知"), notifier=w145) -> ()  [unwired: 1 in, 2 out]
        n93 = Enqueue Element At Opposite End(queue=w146, element=T7 {"命令"="单个写入", {"starting address"=300, "holding register value"=2}} ("元素")) -> ()  [unwired: 2 in, 3 out]
      }
      event "启动": Value Change {
        n94 = event-data() -> ()  [unwired: 1 in, 6 out]
        n95 = flat-sequence {
          tunnel: w148 -> [w149]
          frame #0 {
            n96 = Cancel Notification(0:w149) -> ()  [unwired: 1 in, 3 out]
          }
          frame #1 {
            n97 = call "手动启动选择对话框.vi"() -> ("确定"=w151:bool, "输出簇"=w150:T10)  [unwired: 10 in]
            n98 = case shown="真" w151 {
              tunnel: w150 -> [_ w152]
              frame False {
              }
              frame True {
                n99 = vi-ref "PLC.lvlib:一体站流程自动启动.vi"() -> (w155:refnum<vi>)
                n100 = property class="VI"(reference=w155) -> ("Name"=w154:string, "Exec.State"=w153:T11)  [unwired: 1 in, 2 out]
                n101 = case shown="\"Idle\"" w153 {
                  tunnel: w154 -> [_ w163 _ _]
                  tunnel: w152 -> [_ w157 _ _]
                  frame "Bad", Default {
                  }
                  frame "Idle" {
                    n102 = Open VI Reference(type specifier VI Refnum (for type only)=refnum<vi> refnum, vi path=w163, options=128 ("选项")) -> (vi reference=w161:refnum<vi>, error out=w159:errorcluster)  [unwired: 3 in]
                    n103 = call-by-ref "开始异步调用"(reference=w161, error in=w159, "参数"=w157) -> (reference out=w160:refnum<vi>, error out=w158:errorcluster)  [unwired: 11 in]
                    n104 = Close Reference(reference=w160, error in (no error)=w158) -> ()  [unwired: 1 out]
                  }
                  frame "Run top level" {
                  }
                  frame "Running" {
                    n105 = One Button Dialog(message="流程已启动，无需重复启动！" ("消息")) -> ()  [unwired: 1 in, 1 out]
                  }
                }
              }
            }
          }
        }
      }
      event "单步启动": Value Change {
        n106 = event-data() -> ()  [unwired: 1 in, 6 out]
        n107 = call "单步启动对话框.vi"() -> ("单步启动步骤输出"=w165:u16)  [unwired: 11 in]
        n108 = Bundle By Name(cluster=T2 {"命令"="单个写入", "数据"={"starting address"=301, "holding register value"=0}} ("元素"), "数据.holding register value"=w165) -> (w166:T2)
        n109 = Enqueue Element At Opposite End(queue=w168, element=w166) -> ()  [unwired: 2 in, 3 out]
      }
      event "R101", "R102", "R103", "R104", "R105", "R106", "R107", "R108", "R109", "R100", "R110", "R111", "R112", "R113": Value Change {
        n110 = event-data() -> ()  [unwired: 1 in, 6 out]
        n111 = local read "R101"() -> (w183:i16)
        n112 = local read "R102"() -> (w182:i16)
        n113 = local read "R103"() -> (w181:i16)
        n114 = local read "R104"() -> (w180:i16)
        n115 = local read "R105"() -> (w179:i16)
        n116 = local read "R106"() -> (w178:i16)
        n117 = local read "R107"() -> (w177:i16)
        n118 = local read "R108"() -> (w176:i16)
        n119 = local read "R109"() -> (w174:i16)
        n120 = local read "R110"() -> (w173:i16)
        n121 = local read "R112"() -> (w170:i16)
        n122 = Build Array("R100", w183, w182, w181, w180, w179, w178, w177, w176, w174, w173, "R111", w170, "R113") -> (w172:u16[])
        n123 = Bundle By Name(cluster=T8 {"命令"="多个写入", "数据"={"starting address"=0, "holding register values"=[]}} ("元素"), "数据.starting address"=u16 100, "数据.holding register values"=w172) -> (w184:T8)
        n124 = Enqueue Element At Opposite End(queue=w187, element=w184) -> ()  [unwired: 2 in, 3 out]
      }
      event "R116", "R117", "R118", "R120", "R121", "R122": Value Change {
        n125 = event-data() -> ()  [unwired: 1 in, 6 out]
        n126 = local read "R116"() -> (w194:i16)
        n127 = local read "R117"() -> (w193:i16)
        n128 = local read "R120"() -> (w191:i16)
        n129 = local read "R121"() -> (w190:i16)
        n130 = local read "R122"() -> (w189:i16)
        n131 = Build Array(w194, w193, "R118", i16 0 ("R116"), w191, w190, w189) -> (w195:u16[])
        n132 = Bundle By Name(cluster=T8 {"命令"="多个写入", "数据"={"starting address"=0, "holding register values"=[]}} ("元素"), "数据.starting address"=u16 116, "数据.holding register values"=w195) -> (w197:T8)
        n133 = Enqueue Element At Opposite End(queue=w196, element=w197) -> ()  [unwired: 2 in, 3 out]
      }
      event "R124": Value Change {
        n134 = event-data() -> ("NewVal"=w200:i16)  [unwired: 1 in, 5 out]
        n135 = Build Array(w200) -> (w202:i16[])
        n136 = Bundle By Name(cluster=T8 {"命令"="多个写入", "数据"={"starting address"=0, "holding register values"=[]}} ("元素"), "数据.starting address"=u16 124, "数据.holding register values"=w202) -> (w203:T8)
        n137 = Enqueue Element At Opposite End(queue=w201, element=w203) -> ()  [unwired: 2 in, 3 out]
      }
      event "R101", "R102", "R103", "R104", "R105", "R106", "R107", "R108", "R109", "R117", "R110", "R116", "R112", "R120", "R121", "R122", "R124": Mouse Down {
        n138 = event-data() -> ("CtlRef"=w209:refnum<vi>)  [unwired: 1 in, 7 out]
        n139 = property class="DigNum (严格)"(reference=w209) -> (reference out=w207:refnum<vi>, "Value"=w208:i16)  [unwired: 1 in, 1 out]
        n140 = call "数字键盘.vi"("OldNumber"=w208) -> ("NewNumber"=w206:sgl)
        n141 = property class="DigNum (严格)"(reference=w207, "Val(Sgnl)"=w206) -> ()  [unwired: 1 in, 2 out]
      }
      event "参数设置": Value Change {
        n142 = event-data() -> ()  [unwired: 1 in, 6 out]
        n143 = property on="窗格" class="Pane"("Origin"=T1 {"Horizontal"=0, "Vertical"=628} ("原点")) -> ()  [unwired: 2 in, 2 out]
      }
      event "返回": Value Change {
        n144 = event-data() -> ()  [unwired: 1 in, 6 out]
        n145 = property on="窗格" class="Pane"("Origin"=T1 {"Horizontal"=0, "Vertical"=0} ("原点")) -> ()  [unwired: 2 in, 2 out]
      }
      event "M1", "M2", "V2", "V3", "V4", "V5", "V6", "V7-G", "V7-R", "V8", "V9", "V10", "V11", "V1-G", "V1-R", "V12", "V13", "M4", "M3", "V14": Value Change {
        n146 = event-data() -> ()  [unwired: 1 in, 6 out]
        n147 = Build Array("V1-G", "V1-R", "V2", "V3", "V4", "V5", "V6", "V7-G", "V7-R", "V8", "V9", "V10", "V11", "V12", "V13", "M1", "M2", "M3", "M4", "V14") -> (w228:bool[])
        n148 = Bundle By Name(cluster=T9 {"命令"="线圈写入", "data"={"starting address"=2400, "coil values"=[]}} ("元素"), "data.coil values"=w228) -> (w229:T9)
        n149 = Enqueue Element(queue=w235, element=w229) -> ()  [unwired: 2 in, 3 out]
      }
      event "更新程序": Value Change {
        n150 = event-data() -> ("NewVal"=w236:bool)  [unwired: 1 in, 5 out]
        n151 = case shown="真" w236 {
          tunnel: [cluster{"命令":string, "数据":variant} {"命令"="init", "数据"=variant} ("元素") w243] -> w238
          frame False {
          }
          frame True {
            n152 = Two Button Dialog(message="警告，非专业人士请勿进行此操作！！！\n请确认是否释放串口？" ("消息")) -> (T button?=w242:bool)  [unwired: 2 in]
            n153 = case shown="真" w242 {
              tunnel: [_ cluster{"命令":string, "数据":variant} {"命令"="shutdown", "数据"=variant} ("元素")] -> w243
              frame False {
                n154 = local write "更新程序"(FALSE ("释放串口")) -> ()
              }
              frame True {
              }
            }
          }
        }
        n155 = Flush Queue(queue=w239) -> (queue out=w237:refnum<queue>)  [unwired: 1 in, 2 out]
        n156 = Enqueue Element(queue=w237, element=w238) -> ()  [unwired: 2 in, 3 out]
      }
    }
  }
  n157 = Enqueue Element(queue=w13, element=cluster{"命令":string, "数据":variant} {"命令"="init", "数据"=variant} ("元素"), error in (no error)=w12) -> (queue out=w8:refnum<queue>, error out=w10:errorcluster)  [unwired: 1 in, 1 out]
  n158 = while {
    shift-right: [w251] -> _
    shift-left: _ -> [w253]
    shift-right: [w250] -> _
    shift-left: _ -> [w252]
    shift-right: [w247] -> _
    shift-left: enum16{"open", "read", "write", "close"}."open" -> [w248]
    stop <- FALSE stop-if-true
    # "模块为主站modbustcp地址与其他模块交互\n1氨氮  2总磷 3总氮 4CODMn 5CODCr 10采配水"
    n159 = Wait (ms)(milliseconds to wait=u32 1000 ("等待时间（毫秒）")) -> ()  [unwired: 1 out]
    n160 = case shown="\"write\"" w248 {
      selector: w248 -> [w262 _ _ _]
      tunnel: w253 -> [w256 w268 w279 w285]
      tunnel: w252 -> [w255 w267 w276 w284]
      tunnel: [w259 w265 w275 w285] -> w251
      tunnel: [w258 w266 w274 w287] -> w250
      tunnel: [w261 w271 w280 enum16{"open", "read", "write", "close"}."open"] -> w247
      frame "open", Default {
        n161 = call-dynamic "Shutdown.vi"("error in"=w255, "Modbus slave in"=w256) -> ("error out"=w254:errorcluster)  [unwired: 9 in]
        n162 = call <vilib>:"Clear Errors.vi"("error in (no error)"=w254) -> ("error out"=w257:errorcluster)  [unwired: 5 in, 1 out]
        n163 = call-poly <vilib>:"Create Modbus Instance.vi"("error in"=w257, "port (502)"=u16 10) -> ("error out"=w258:errorcluster, "TCP slave instance"=w259:refnum<class "Modbus Slave.lvclass">)  [unwired: 8 in]
        n164 = case shown="无错误" w258 {
          tunnel: w262 -> [_ w264]
          tunnel: [enum16{"open", "read", "write", "close"}."write" w264] -> w261
          frame No Error {
          }
          frame Error {
          }
        }
      }
      frame "read" {
        n165 = call-dynamic <vilib>:"Read Holding Registers.vi"("error in"=w267, "number of inputs"=u16 1, "starting address"=u16 257, "Modbus slave in"=w268) -> ("error out"=w266:errorcluster, "Modbus slave out"=w265:refnum<class "Modbus Slave.lvclass">)  [unwired: 5 in, 1 out]
        n166 = case shown="无错误" w266 {
          tunnel: [enum16{"open", "read", "write", "close"}."write" enum16{"open", "read", "write", "close"}."close"] -> w271
          frame No Error {
          }
          frame Error {
          }
        }
      }
      frame "write" {
        n167 = local read "Registers"() -> (w277:u16[])
        n168 = call-dynamic "Write Multiple Holding Registers.vi"("error in"=w276, "registers to write"=w277, "starting address"=u16 0, "Modbus slave in"=w279) -> ("error out"=w274:errorcluster, "Modbus slave out"=w275:refnum<class "Modbus Slave.lvclass">)  [unwired: 6 in]
        n169 = case shown="无错误" w274 {
          tunnel: [enum16{"open", "read", "write", "close"}."write" enum16{"open", "read", "write", "close"}."close"] -> w280
          frame No Error {
          }
          frame Error {
          }
        }
      }
      frame "close" {
        n170 = call-dynamic "Shutdown.vi"("error in"=w284, "Modbus slave in"=w285) -> ("error out"=w283:errorcluster)  [unwired: 9 in]
        n171 = call <vilib>:"Clear Errors.vi"("error in (no error)"=w283) -> ("error out"=w287:errorcluster)  [unwired: 5 in, 1 out]
      }
    }
  }
  n172 = while {
    tunnel: w8 -> [w292]
    tunnel: w10 -> [w291]
    shift-right: [w295] -> w5
    shift-left: refnum<class "MB_Master.lvclass"> refnum ("MB session in") -> [w294]
    tunnel: errorcluster {"status"=FALSE, "code"=0, "source"=""} ("error out") -> [w293]
    tunnel: [w290] -> w6
    stop <- FALSE stop-if-true
    n173 = case shown="无错误" w293 {
      selector: w293 -> [w301 w511]
      tunnel: [w304 w510] -> w295
      tunnel: w294 -> [w303 w512]
      tunnel: [w302 w508] -> w290
      tunnel: w292 -> [w298 w507]
      tunnel: w291 -> [w297 _]
      tunnel: [w299 _] -> _
      frame No Error {
        n174 = Dequeue Element(queue=w298, error in (no error)=w297) -> (element=w296:cluster{"命令":string, "数据":variant})  [unwired: 1 in, 3 out]
        n175 = Unbundle By Name(w296) -> ("命令"=w300:string)
        n176 = case shown="\"shutdown\"" w300 {
          tunnel: [w306 w319 w329 w447 w459 w469 w479 w494] -> w304
          tunnel: w303 -> [w306 w321 w413 w452 w462 w472 w482 w494]
          tunnel: [w305 w320 w330 w446 w460 w470 w480 w485] -> w302
          tunnel: w301 -> [w305 w323 w416 w451 w461 w471 w481 w490]
          tunnel: [_ _ _ _ _ _ _ TRUE] -> w299
          tunnel: w296 -> [_ _ _ _ w458 w468 w478 _]
          frame "idle", Default {
          }
          frame "init" {
            w310 = refnum<visa-resource-name> "COM3" ("VISA resource name")
            n177 = call-dynamic "Close Session.vi"("error in (no error)"=w323, "MB session in"=w321) -> ("error out"=w322:errorcluster)  [unwired: 9 in]
            n178 = call <vilib>:"Clear Errors.vi"("error in (no error)"=w322) -> ("error out"=w308:errorcluster)  [unwired: 5 in, 1 out]
            n179 = call-poly "VISA Configure Serial Port"("VISA resource name"=w310, "baud rate (9600)"=u32 115200, "error in (no error)"=w308) -> ("VISA resource name out"=w315:refnum<visa-resource-name>, "error out"=w314:errorcluster)  [unwired: 11 in]
            n180 = VISA Write(VISA resource name=w315, write buffer="\u0002004701R04047560A5B\u0003" ("写入缓冲区"), error in (no error)=w314) -> (VISA resource name out=w313:refnum<visa-resource-name>, error out=w312:errorcluster)  [unwired: 1 out]
            n181 = VISA Close(VISA resource name=w313, error in (no error)=w312) -> (error out=w307:errorcluster)
            n182 = call <vilib>:"Open Serial Session.vi"("Mode (RTU)"=enum16{"RTU", "ASCII"}."RTU", "Error in"=w307, "Slave ID"=u8 10, "Serial Config"=T12 {"baud rate (bps)"=115200, "stop bits"=10, "parity"=0, "flow control"=0, "timeout"=500, "retries"=1}, "VISA Resource"=w310) -> ("Error out"=w320:errorcluster, "MB_Serial session"=w319:refnum<class "MB_Master_Serial.lvclass">)  [unwired: 5 in]
            n183 = Unbundle By Name(w320) -> ("status"=w324:bool)
            n184 = call "对话框信息"("Enable"=w324) -> ()  [unwired: 9 in, 2 out]
          }
          frame "读状态" {
            # "压力传感器\n4-20  mA \n \n0-8191\n\n0-1MPA"
            n185 = call <vilib>:"Read Holding Registers.vi"("error in (no error)"=w416, "quantity"=u16 57 ("number of holding registers"), "starting address"=u16 0, "MB session in"=w413) -> ("error out"=w411:errorcluster, "Registers"=w355:u16[], "MB session out"=w412:refnum<class "MB_Master.lvclass">)  [unwired: 5 in]
            "Registers" <- w355
            n186 = Array To Cluster(array=w355) -> (cluster=w334:T16)
            n187 = Array Subset(array=w355, index=48 ("索引")) -> (w381:u16[])  [unwired: 1 in]
            n188 = Index Array(array=w355, index #1=13 ("索引")) -> (element #1=→"数值":u16, element #2=→"数值 2":u16, element #3=→"数值 3":u16, element #4=→"数值 4":u16, element #5=→"数值 5":u16, element #6=→"数值 6":u16, element #7=→"数值 7":u16, element #8=→"数值 8":u16, element #9=→"数值 9":u16, element #10=→"数值 10":u16, element #11=→"数值 11":u16, element #12=→"数值 12":u16, element #13=→"数值 13":u16, element #14=→"数值 14":u16, element #15=→"数值 15":u16, element #16=→"数值 16":u16, element #17=→"数值 17":u16, element #18=→"数值 18":u16, element #19=→"数值 19":u16)  [unwired: 18 in]
            n189 = global write "采配水全局变量.vi" "状态"(w334) -> ()
            n190 = call <vilib>:"Read Holding Registers.vi"("error in (no error)"=w411, "quantity"=u16 6 ("number of holding registers"), "starting address"=u16 3840, "MB session in"=w412) -> ("error out"=w407:errorcluster, "Registers"=w384:u16[], "MB session out"=w408:refnum<class "MB_Master.lvclass">)  [unwired: 5 in]
            n191 = To Word Integer(number=w384) -> (16bit integer=w383:i16[])
            n192 = call "FATEK_HexToString.vi"("数组"=w381) -> ("STRING"=w380:string[])  [unwired: 10 in]
            n193 = Array To Cluster(array=w384) -> (cluster=w423:T17)
            n194 = global write "采配水全局变量.vi" "AD"(w423) -> ()
            n195 = Index Array(array=w380) -> (element=→"采配水版本号":string)  [unwired: 1 in]
            n196 = call <vilib>:"Read Coils.vi"("error in (no error)"=w407, "quantity"=u16 32 ("number of coils"), "starting address"=u16 0, "MB session in"=w408) -> ("error out"=w403:errorcluster, "Coils"=w388:bool[], "MB session out"=w404:refnum<class "MB_Master.lvclass">)  [unwired: 5 in]
            n197 = global write "采配水全局变量.vi" "输出状态"(w388) -> ()
            n198 = Index Array(array=w388, index #20=31 ("索引")) -> (element #1=w362:bool, element #2=w378:bool, element #3=w377:bool, element #4=w376:bool, element #5=w375:bool, element #6=w374:bool, element #7=w373:bool, element #8=w369:bool, element #9=w368:bool, element #10=w367:bool, element #11=w366:bool, element #12=w365:bool, element #13=w364:bool, element #14=w361:bool, element #15=w360:bool, element #16=w359:bool, element #17=w358:bool, element #18=w357:bool, element #19=w356:bool, element #20=w332:bool)  [unwired: 19 in]
            n199 = formula code="float AD0,AD1,AD2,AD3,AD4,AD5,AD6;\n\nAD0 = IN[0]*140/6553-75;\nAD1 = IN[1]/65.53-25;\nAD2 = (IN[2]/65.53-25)/100;\nAD3 = IN[3]*30/8191;\nAD4 = IN[4]*30/8191;\nAD5 = IN[5]*30/8191;"("IN"=w383) -> ("AD0"=w421:dbl, "AD1"=w420:dbl, "AD2"=w363:dbl, "AD3"=w419:dbl, "AD4"=w418:dbl, "AD5"=w417:dbl)
            "压力传感器" <- w363
            n200 = call <vilib>:"Read Coils.vi"("error in (no error)"=w403, "quantity"=u16 16 ("number of coils"), "starting address"=u16 1000, "MB session in"=w404) -> ("error out"=w399:errorcluster, "Coils"=w395:bool[], "MB session out"=w400:refnum<class "MB_Master.lvclass">)  [unwired: 5 in]
            n201 = local write "V1-G"(w362) -> ()
            n202 = local write "V1-R"(w378) -> ()
            n203 = local write "V2"(w377) -> ()
            n204 = local write "V3"(w376) -> ()
            n205 = local write "V4"(w375) -> ()
            n206 = local write "V5"(w374) -> ()
            n207 = local write "V6"(w373) -> ()
            n208 = local write "V7-G"(w369) -> ()
            n209 = local write "V7-R"(w368) -> ()
            n210 = local write "V8"(w367) -> ()
            n211 = local write "V9"(w366) -> ()
            n212 = local write "V10"(w365) -> ()
            n213 = local write "V11"(w364) -> ()
            n214 = local write "V12"(w361) -> ()
            n215 = local write "V13"(w360) -> ()
            n216 = local write "M1"(w359) -> ()
            n217 = local write "M2"(w358) -> ()
            n218 = local write "M3"(w357) -> ()
            n219 = local write "M4"(w356) -> ()
            n220 = local write "V14"(w332) -> ()
            n221 = global write "采配水全局变量.vi" "输入状态"(w395) -> ()
            n222 = Bundle(w421, w420, w363, w419, w418, w417) -> (w422:cluster{dbl, dbl, dbl, dbl, dbl, dbl})  [unwired: 1 in]
            n223 = Index Array(array=w395) -> (element #1=→"X0":bool, element #2=→"X1":bool, element #3=→"X2":bool, element #4=→"X3":bool, element #5=→"X4":bool, element #6=→"X5":bool, element #7=→"X6":bool, element #8=→"X7":bool, element #9=→"X8":bool, element #10=→"X9":bool, element #11=→"X10":bool, element #12=→"X11":bool)  [unwired: 12 in]
            n224 = global write "采配水全局变量.vi" "转换值"(w422) -> ()
            n225 = call <vilib>:"Read Coils.vi"("error in (no error)"=w399, "quantity"=u16 16 ("number of coils"), "starting address"=u16 2500, "MB session in"=w400) -> ("error out"=w330:errorcluster, "Coils"=w396:bool[], "MB session out"=w331:refnum<class "MB_Master.lvclass">)  [unwired: 5 in]
            n226 = global write "采配水全局变量.vi" "报警簇"(w396) -> ()
            n227 = call <vilib>:"Read Coils.vi"("quantity"=u16 1, "starting address"=u16 2800, "MB session in"=w331) -> ("Coils"=w326:bool[], "MB session out"=w329:refnum<class "MB_Master.lvclass">)  [unwired: 6 in, 1 out]
            n228 = Index Array(array=w326) -> (element=w325:bool)  [unwired: 1 in]
            n229 = global write "采配水全局变量.vi" "看门狗启用"(w325) -> ()
          }
          frame "读参数" {
            n230 = call <vilib>:"Read Holding Registers.vi"("error in (no error)"=w451, "quantity"=u16 25 ("number of holding registers"), "starting address"=u16 100, "MB session in"=w452) -> ("error out"=w446:errorcluster, "Registers"=w448:u16[], "MB session out"=w447:refnum<class "MB_Master.lvclass">)  [unwired: 5 in]
            n231 = Array To Cluster(array=w448) -> (cluster=w436:T18)
            n232 = global write "采配水全局变量.vi" "参数设置"(w436) -> ()
            n233 = Unbundle(w436) -> ("Registers[0]"=w435:u16, "Registers[1]"=→"R101":u16, "Registers[2]"=→"R102":u16, "Registers[3]"=→"R103":u16, "Registers[4]"=→"R104":u16, "Registers[5]"=→"R105":u16, "Registers[6]"=→"R106":u16, "Registers[7]"=→"R107":u16, "Registers[8]"=→"R108":u16, "Registers[9]"=→"R109":u16, "Registers[10]"=→"R110":u16, "Registers[11]"=w432:u16, "Registers[12]"=→"R112":u16, "Registers[13]"=w430:u16, "Registers[16]"=→"R116":u16, "Registers[17]"=→"R117":u16, "Registers[18]"=w428:u16, "Registers[20]"=→"R120":u16, "Registers[21]"=→"R121":u16, "Registers[22]"=→"R122":u16, "Registers[24]"=→"R124":u16)  [unwired: 4 out]
            n234 = local write "R100"(w435) -> ()
            n235 = local write "R111"(w432) -> ()
            n236 = local write "R113"(w430) -> ()
            n237 = local write "R118"(w428) -> ()
          }
          frame "多个写入" {
            n238 = Unbundle By Name(w458) -> ("数据"=w457:variant)
            n239 = Variant To Data(type=T13 {"starting address"=0, "holding register values"=[]}, Variant=w457) -> (data=w455:T13)  [unwired: 1 in, 1 out]
            n240 = Unbundle By Name(w455) -> ("starting address"=w454:u16, "holding register values"=w453:u16[])
            n241 = call <vilib>:"Write Multiple Registers.vi"("error in (no error)"=w461, "values"=w453, "starting address"=w454, "MB session in"=w462) -> ("error out"=w460:errorcluster, "MB session out"=w459:refnum<class "MB_Master.lvclass">)  [unwired: 6 in]
          }
          frame "单个写入" {
            n242 = Unbundle By Name(w468) -> ("数据"=w467:variant)
            n243 = Variant To Data(type=T14 {"starting address"=0, "holding register value"=0}, Variant=w467) -> (data=w465:T14)  [unwired: 1 in, 1 out]
            n244 = Unbundle By Name(w465) -> ("starting address"=w464:u16, "holding register value"=w463:u16)
            n245 = call <vilib>:"Write Single Register.vi"("error in (no error)"=w471, "value"=w463, "address"=w464, "MB session in"=w472) -> ("error out"=w470:errorcluster, "MB session out"=w469:refnum<class "MB_Master.lvclass">)  [unwired: 6 in]
          }
          frame "线圈写入" {
            n246 = Unbundle By Name(w478) -> ("数据"=w477:variant)
            n247 = Variant To Data(type=T15 {"starting address"=0, "coil values"=[]}, Variant=w477) -> (data=w475:T15)  [unwired: 1 in, 1 out]
            n248 = Unbundle By Name(w475) -> ("starting address"=w474:u16, "coil values"=w473:bool[])
            n249 = call <vilib>:"Write Multiple Coils.vi"("error in (no error)"=w481, "values"=w473, "starting address"=w474, "MB session in"=w482) -> ("error out"=w480:errorcluster, "MB session out"=w479:refnum<class "MB_Master.lvclass">)  [unwired: 6 in]
          }
          frame "shutdown" {
            n250 = call <vilib>:"Write Single Register.vi"("error in (no error)"=w490, "value"=u16 0, "address"=u16 4047, "MB session in"=w494) -> ("error out"=w489:errorcluster, "MB session out"=w493:refnum<class "MB_Master.lvclass">)  [unwired: 6 in]
            n251 = call-dynamic "Close Session.vi"("error in (no error)"=w489, "MB session in"=w493) -> ("error out"=w495:errorcluster)  [unwired: 9 in]
            n252 = call "文件对话框"("start path"=path "D:/SRC", "pattern (all files)"="*.pdw", "pattern label"="PLC") -> ("selected path"=w488:path, "cancelled"=w486:bool)  [unwired: 9 in, 2 out]
            n253 = call <vilib>:"Clear Errors.vi"("error in (no error)"=w495) -> ("error out"=w485:errorcluster)  [unwired: 5 in, 1 out]
            n254 = case shown="假" w486 {
              tunnel: w488 -> [w501 _]
              tunnel: w485 -> [_ _]
              frame False {
                n255 = Path To String(path=w501) -> (string=w498:string)
                n256 = Format Into String(format string="  - \"%s\"" ("格式字符串"), initial string="\"C:\\Program Files\\Fatek\\WinProladder\\WProlad.exe\"" ("command line"), w498) -> (resulting string=w499:string)  [unwired: 1 in, 1 out]
                n257 = call <vilib>:"System Exec.vi"("command line"=w499) -> ("error out"=w502:errorcluster)  [unwired: 7 in, 3 out]
                n258 = case shown="错误" w502 {
                  tunnel: w498 -> [_ w505]
                  frame No Error {
                  }
                  frame Error {
                    n259 = Format Into String(format string="  - \"%s\"" ("格式字符串"), initial string="\"C:\\Program Files (x86)\\Fatek\\WinProladder\\WProlad.exe\"" ("command line"), w505) -> (resulting string=w503:string)  [unwired: 1 in, 1 out]
                    n260 = call <vilib>:"System Exec.vi"("command line"=w503) -> ()  [unwired: 7 in, 4 out]
                  }
                }
              }
              frame True {
              }
            }
          }
        }
      }
      frame Error {
        n261 = Unbundle By Name(w511) -> ("code"=w513:i32)
        n262 = case shown="-1073807343" w513 {
          tunnel: w512 -> [w515 w519]
          tunnel: w511 -> [w514 w521]
          tunnel: [w514 w520] -> w509
          tunnel: [w515 w519] -> w510
          tunnel: w507 -> [_ w518]
          frame Default {
          }
          frame -1073807343 {
            n263 = Flush Queue(queue=w518) -> (queue out=w517:refnum<queue>)  [unwired: 1 in, 2 out]
            n264 = call-dynamic "Close Session.vi"("error in (no error)"=w521, "MB session in"=w519) -> ("error out"=w520:errorcluster)  [unwired: 9 in]
            n265 = disable-structure shown="禁用" {
              disable-tunnel: w517 -> [w522 _]
              frame Disabled {
                n266 = Enqueue Element At Opposite End(queue=w522, element=cluster{"命令":string, "数据":variant} {"命令"="init", "数据"=variant} ("元素")) -> ()  [unwired: 2 in, 3 out]
              }
              frame Enabled {
              }
            }
            n267 = Wait (ms)(milliseconds to wait=u32 2000 ("等待时间（毫秒）")) -> ()  [unwired: 1 out]
          }
        }
        n268 = call <vilib>:"Clear Errors.vi"("error in (no error)"=w509) -> ("error out"=w508:errorcluster)  [unwired: 5 in, 1 out]
      }
    }
    n269 = Unbundle By Name(w290) -> ("status"=→"通讯故障":bool)
  }
  n270 = property on="多列列表框" class="MCListbox (严格)"("ItemNames"=string[][] [["待机"], ["初始化"], ["水样润洗"], ["一级水样池进样"], ["二级水样池进样"], ["一级补充水样"], ["沉淀配水"], ["反冲洗"], ["采样池储水"], ["结束"]] ("项名")) -> ()  [unwired: 2 in, 2 out]
  n271 = call-dynamic "Close Session.vi"("error in (no error)"=w6, "MB session in"=w5) -> ()  [unwired: 9 in, 1 out]
